vi "Demo_Main-Administrator-an.vi"() -> ()   [LabVIEW 2010]
uses:
  ControlCAN/ControlCAN.llb/DevType.ctl
  ControlCAN/ControlCAN.llb/CAN Channel.ctl
  ControlCAN/ControlCAN.llb/InitFlag.ctl
  ControlCAN/ControlCAN.llb/Mode.ctl
  ControlCAN/ControlCAN.llb/Fliter.ctl
  ControlCAN/ControlCAN.llb/VCI_CAN_OBJ.ctl
  ControlCAN/ControlCAN.llb/VCI_INIT_CONFIG.ctl
  ControlCAN/ControlCAN.llb/Return Val.ctl
  ControlCAN/ControlCAN.lvlib
panel:
  in  "T4":u16
  in  "W4":u16
  in  "W3":u16
  out "W4":u16
  in  "W4_R":bool
  in  "W4_W":bool
  in  "W3_R":bool
  out "W3":u16
  in  "W3_W":bool
  out "W2":u16
  in  "W2_R":bool
  in  "W2_W":bool
  in  "W2":u16
  in  "W1_R":bool
  in  "W1":u16
  out "W1":u16
  in  "W1_W":bool
  in  "电机自动校准":string(combo)="0"
  in  "电机校准_W":bool
  in  "T4_R":bool
  out "T4":u16
  in  "T4_W":bool
  in  "减速度_R":bool
  in  "减速度":dbl format="%#.6f"
  out "减速度_回":dbl format="%#.6f"
  in  "减速度_W":bool
  out "版本号":dbl format="%_3f"
  in  "看门狗周期_R":bool
  in  "看门狗周期":u16
  out "看门狗周期_回":u16
  in  "看门狗周期_W":bool
  in  "看门狗_W":bool
  in  "看门狗":string(combo)="开启"
  in  "监测周期_R":bool
  in  "监测周期":u16
  out "监测周期_回":u16
  in  "监测周期_W":bool
  out "ERRO7":bool
  out "ERRO6":bool
  out "ERRO5":bool
  out "ERRO4":bool
  out "ERRO3":bool
  out "高温":bool
  out "高压":bool
  out "低压":bool
  out "warn7":bool
  out "warn6":bool
  out "warn5":bool
  out "warn4":bool
  out "warn3":bool
  out "高温":bool
  out "warn1":bool
  out "warn0":bool
  out "温度":dbl format="%#.6f"
  out "转速":dbl(graph)
  out "CAN ID":u8 format="%x"
  out "数组":u8[](array[numeric]) format="%x"
  in  "DATA_SAVE_W":bool
  out "T3":u16
  out "T2":u16
  in  "T3_R":bool
  in  "T2_R":bool
  in  "T3_W":bool
  in  "T2_W":bool
  in  "T3":u16
  in  "T2":u16
  in  "T1_R":bool
  in  "T1":u16
  out "T1":u16
  in  "T1_W":bool
  out "Sin":i32
  out "Cosin":i32
  in  "加速度_R":bool
  in  "加速度":dbl format="%#.6f"
  out "加速度_回":dbl format="%#.6f"
  in  "加速度_W":bool
  in  "速度环KI_R":bool
  in  "W_EN_R":bool
  in  "速度环KI":dbl format="%#.6f"
  out "速度环KI_回":dbl format="%#.6f"
  in  "速度环KI_W":bool
  in  "过载诊断使能":i8
  out "功率使能":i8
  in  "W_EN_W":bool
  in  "I_EN_R":bool
  in  "Direction_R":bool
  in  "电流诊断使能":i8
  out "电流使能":i8
  in  "I_EN_W":bool
  in  "方向":u16
  out "方向":i8
  in  "Direction_W":bool
  out "波形图表3":dbl(graph)
  out "波形图表2":dbl(graph)
  out "波形图表1":dbl(graph)
  out "sCnt":u32 caption="处理统计"
  out "模式_回":string(combo)="00"
  in  "模式_R":bool
  in  "设定电流_R":bool
  in  "设定位置_R":bool
  in  "设定速度_R":bool
  in  "存储路径":path
  in  "保存":bool
  out "保存_S":bool
  in  "模式_W":bool
  in  "模式":string(combo)="00"
  in  "设定电流":dbl format="%#.6f"
  out "设定电流_回":dbl format="%#.6f"
  in  "设定电流_W":bool
  in  "设定位置":dbl format="%#.6f"
  out "设定位置_回":dbl format="%#.6f"
  in  "设定位置_W":bool
  in  "设定速度":dbl format="%#.1f"
  out "设定速度_回":dbl format="%#.6f"
  in  "设定速度_W":bool
  in  "监测_W":bool
  in  "监测":string(combo)="30"
  out "电机ID_R":u32
  in  "Clear":bool
  out "Ualfa":dbl format="%#.6f"
  out "Ubate":dbl format="%#.6f"
  out "Uq":dbl format="%#.6f"
  out "Ud":dbl format="%#.6f"
  out "PWM1":u16
  out "PWM2":u16
  out "PWM3":u16
  out "sector":u8
  out "Iqnow":dbl
  out "Idnow":dbl
  out "Ialfa":dbl
  out "Ibeta":dbl
  out "A电流":dbl
  out "C电流":dbl
  out "B电流":dbl
  out "供电电压":dbl
  out "机械角度":dbl format="%.2f"
  out "电气角度":dbl
  out "转速":dbl
  out "CAN STD_ID":u32 format="%x"
  in  "电机ID":string(combo)="00"
  in  "电机ID_W":bool
  out "RecvCnt":u32 caption="接收统计"
  out "SendCnt":u32 caption="发送统计"
  in  "Format":u8(ring) items=["标准帧", "扩展帧"]
  in  "Type":u8(ring) items=["数据帧", "远程帧"]
  in  "Data":string="00 01 02 03 04 05 06 07"
  in  "ID":u32=291 format="0x%x"
  in  "Send":bool
  in  "RcvEnable":bool=TRUE
  out "Open":bool
  in  "Fliter":T1=1 items=["接收所有类型"=1, "只接收标准帧"=2, "只接收扩展帧"=3]
  in  "kBaudRate":u8(ring)=12 caption="波特率" items=["5k bps"=1, "10k bps"=2, "20k bps"=3, "40k bps"=4, "50k bps"=5, "80k bps"=6, "100k bps"=7, "125k bps"=8, "200k bps"=9, "250k bps"=10, "400k bps"=11, "500k bps"=12, "666k bps"=13, "800k bps"=14, "1000k bps"=15, "33.33k bps"=16, "66.66k bps"=17, "83.33k bps"=18]
  in  "Mode":T2 caption="工作模式" items=["正常工作", "仅侦听模式", "自测模式（环回）"]
  in  "InitFlag":T3 caption="初始化参数" items=["使用Flash参数", "使用界面设置参数"]
  in  "AccMask":u32=4294967295 caption="接收屏蔽码" format="%08x"
  in  "AccCode":u32 caption="接收过滤码" format="%08x"
  in  "Close":bool
  in  "Open":bool
  in  "Channel":T4 caption="CAN通道" items=["通道1", "通道2"]
  in  "DevType":T5=3 caption="设备类型" items=["USB-CAN"=2, "USB-CAN2"=3]
  # "发送指令帧包"
  # "CAN\n  ID"
  # "DATA"
  # "DATA"
  # "DATA"
  # "0"
  # "1"
  # "7"
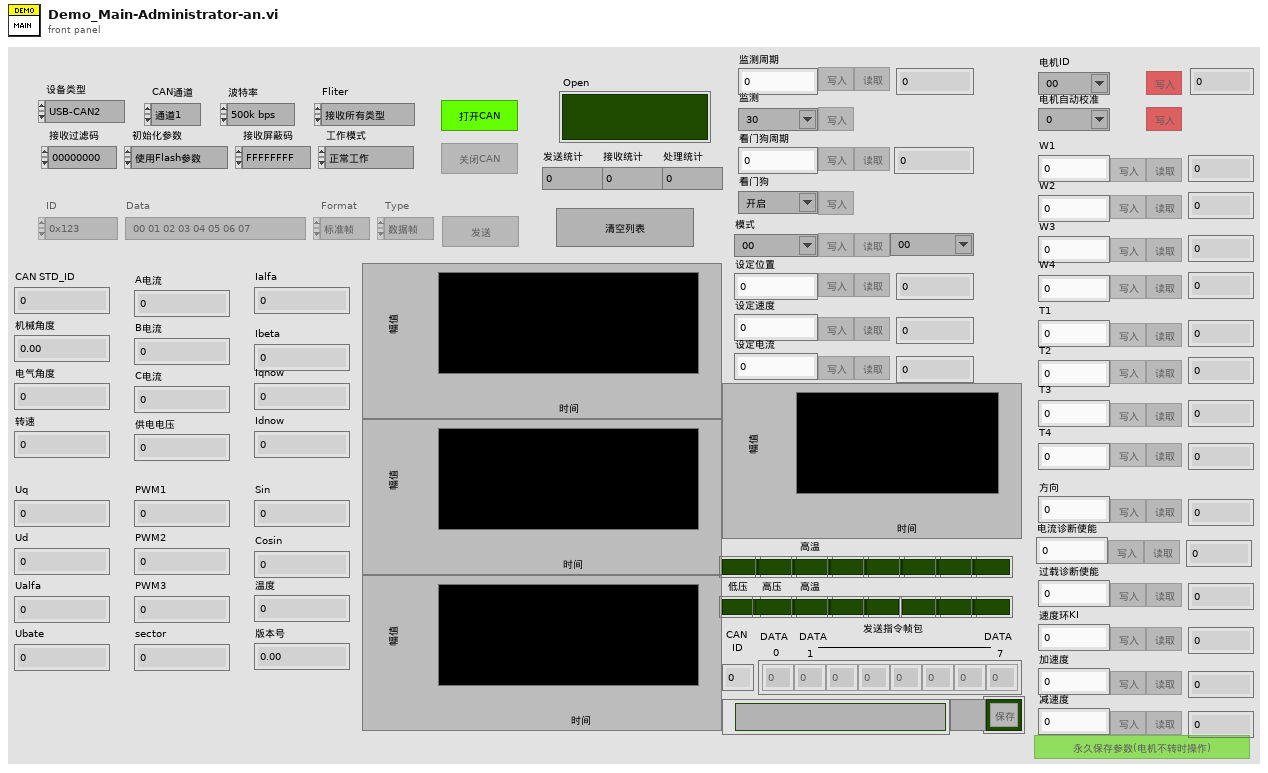
[diagram p1: front panel]
types:
  T1 = typedef "ControlCAN.lvlib/Fliter.ctl" = u8
  T2 = typedef "ControlCAN.lvlib/Mode.ctl" = u8
  T3 = typedef "ControlCAN.lvlib/InitFlag.ctl" = u32
  T4 = typedef "ControlCAN.lvlib/CAN Channel.ctl" = u32
  T5 = typedef "ControlCAN.lvlib/DevType.ctl" = u32
  T6 = typedef "ControlCAN.lvlib/VCI_CAN_OBJ.ctl" = cluster{"ID":u32, "TimeStamp":u32, "TimeFlag":u8, "SendType":u8, "RemoteFlag":u8, "ExternFlag":u8, "DataLen":u8, "Data":u8[], "Reserved":u8[]}
  T7 = cluster{"Type":enum16{"接收", "发送"}, "Channel":T4, "Time":timestamp, "VCI_CAN_OBJ":T6}[]
  T8 = typedef "ControlCAN.lvlib/VCI_INIT_CONFIG.ctl" = cluster{"AccCode":u32, "AccMask":u32, "InitFlag":T3, "Fliter":T1, "Timing0":u8, "Timing1":u8, "Mode":T2}
  T9 = cluster{"DevType":T5, "DevIndex":u32, "CanIndex":T4, "VCI_INIT_CONFIG":T8}
  T10 = typedef "ControlCAN.lvlib/Return Val.ctl" = i32
  T11 = enum16{"open", "replace", "create", "open or create", "replace or create", "replace or create with confirmation"}
  T12 = cluster{"[0]":cluster{"Type":enum16{"接收", "发送"}, "Channel":T4, "Time":timestamp, "VCI_CAN_OBJ":T6}}
  T13 = cluster{"Type":enum16{"接收", "发送"}, "Channel":T4, "Time":timestamp, "VCI_CAN_OBJ":T6}
  T14 = cluster{"Data[0]":u8, "Data[1]":u8, "Data[2]":u8, "Data[3]":u8, "Data[4]":u8, "Data[5]":u8, "Data[6]":u8, "Data[7]":u8}
  T15 = cluster{"Boolean array[0]":bool, "Boolean array[1]":bool, "Boolean array[2]":bool, "Boolean array[3]":bool, "Boolean array[4]":bool, "Boolean array[5]":bool, "Boolean array[6]":bool, "Boolean array[7]":bool}
  T16 = enum32{"invalid app kind", "Development System", "Run Time System", "Student Edition", "Embedded LabVIEW", "Evaluation", "Custom"}
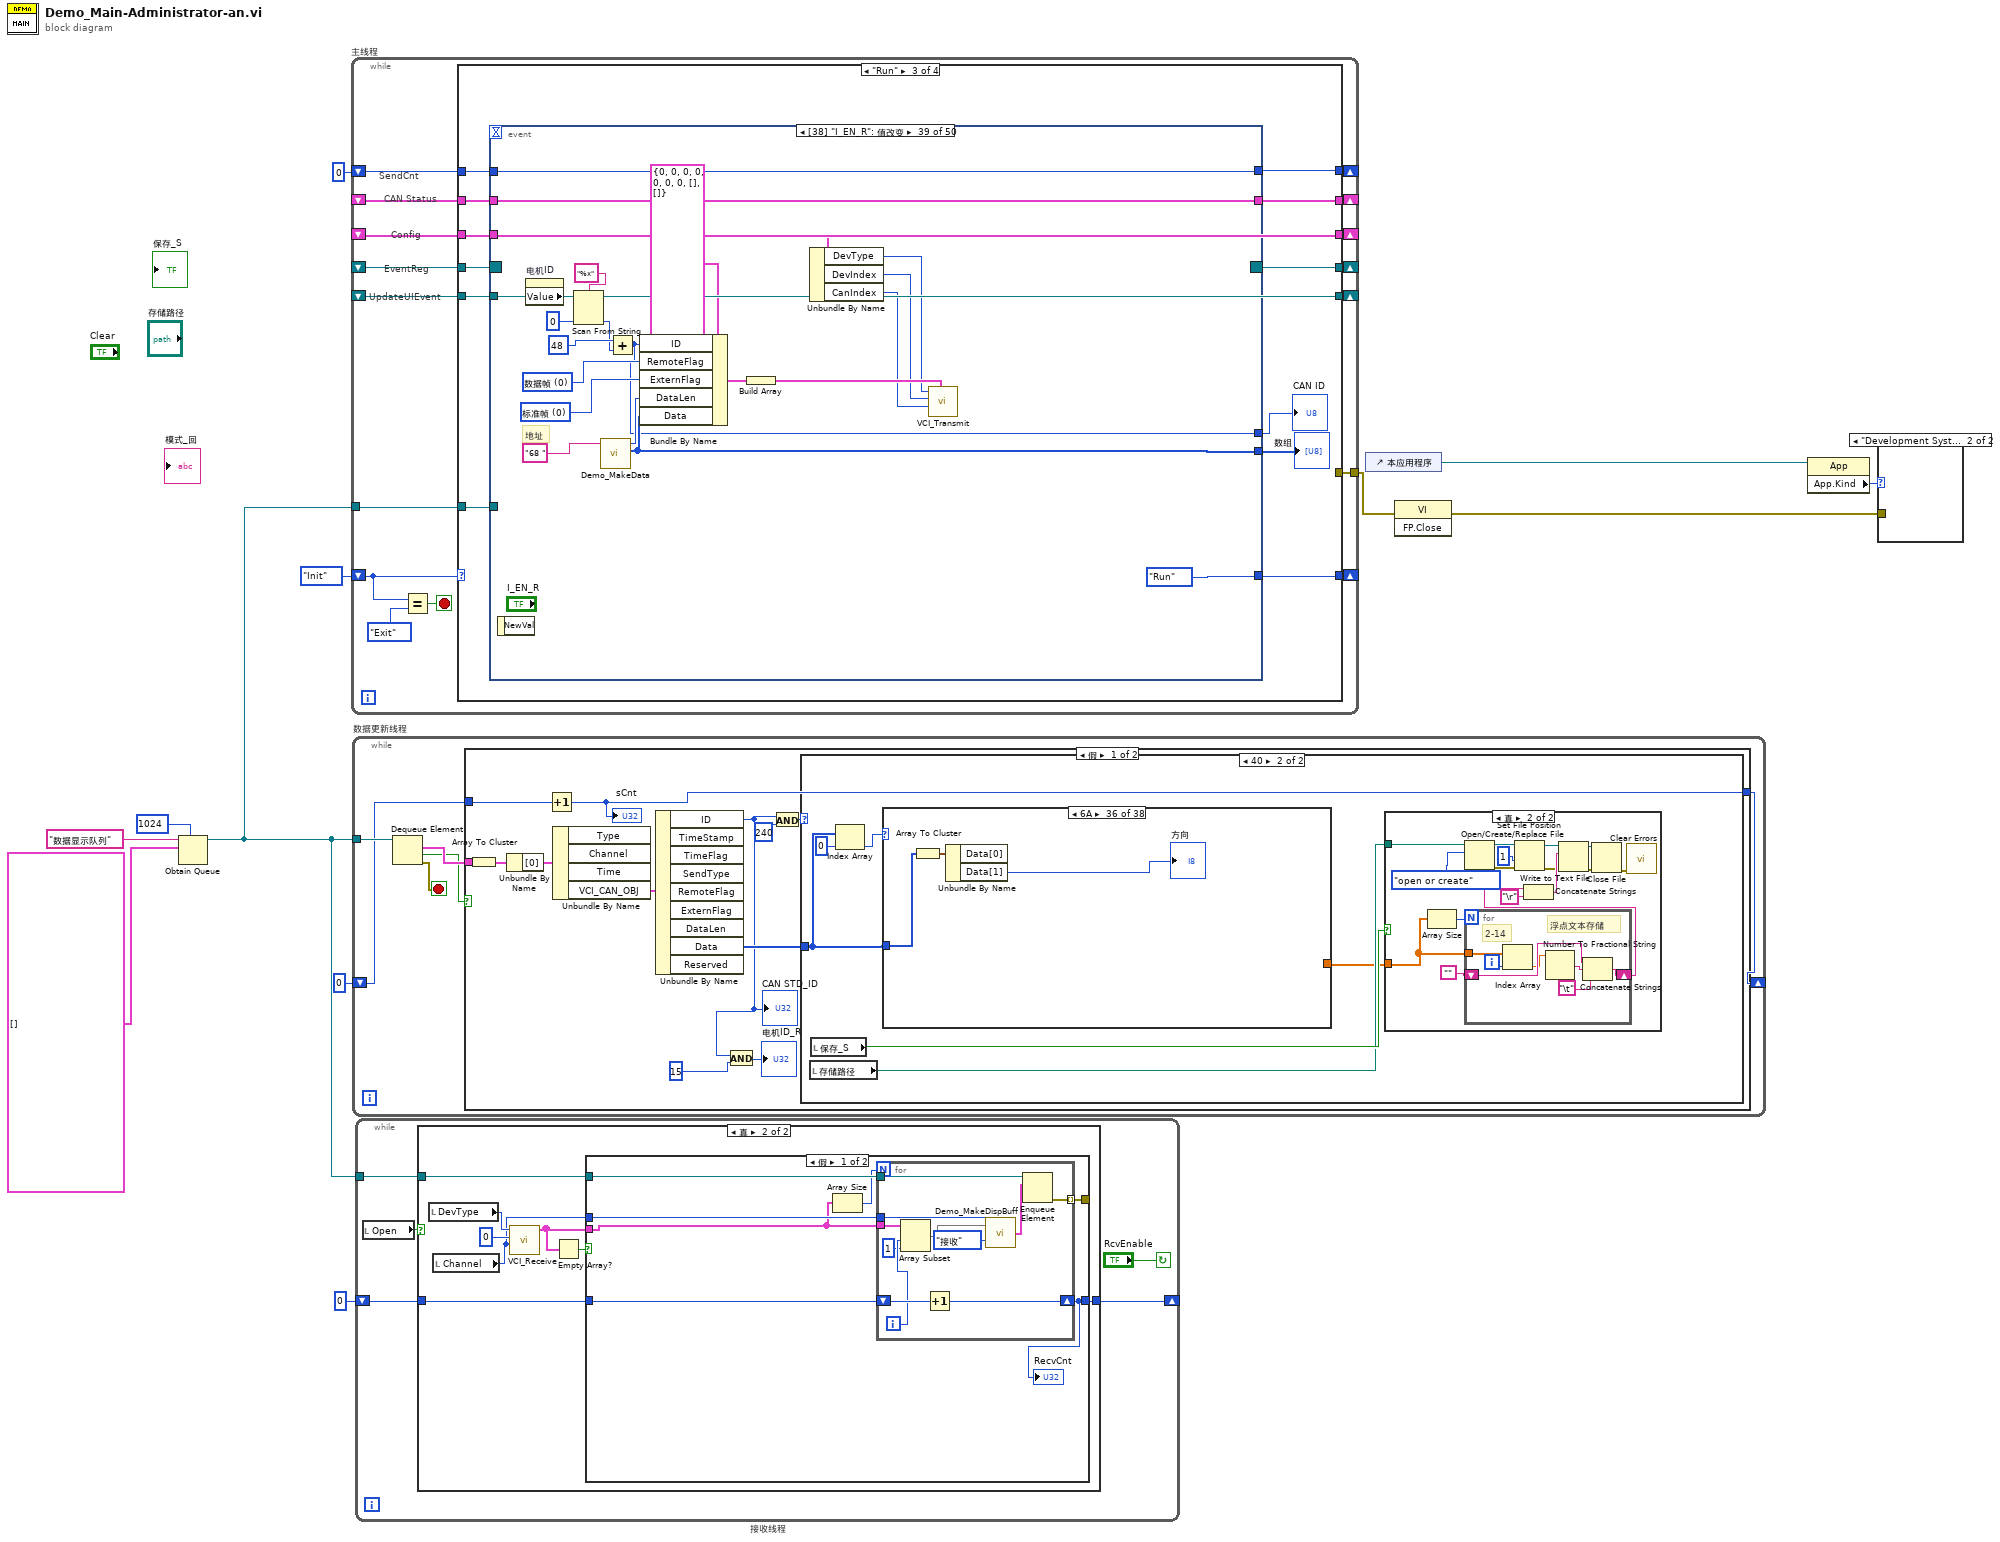
[diagram p0: block diagram]
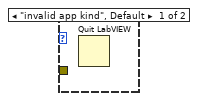
[diagram p2: hidden frame]
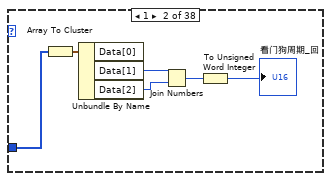
[diagram p6: hidden frame]
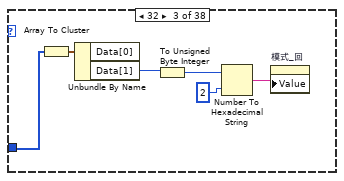
[diagram p7: hidden frame]
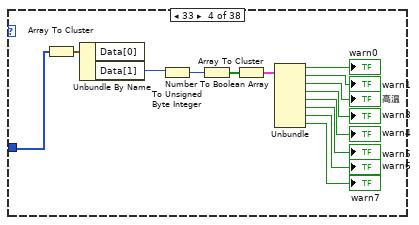
[diagram p8: hidden frame]
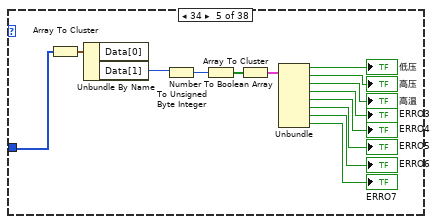
[diagram p9: hidden frame]
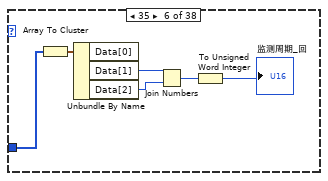
[diagram p10: hidden frame]
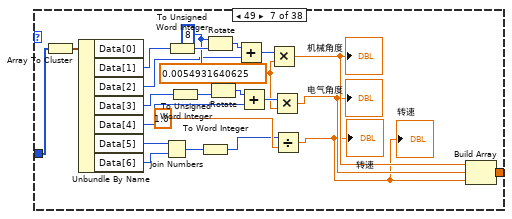
[diagram p11: hidden frame]
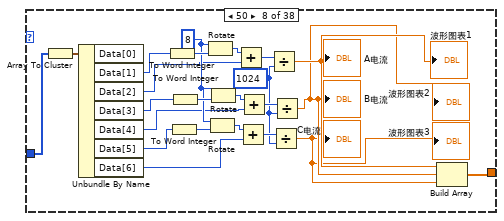
[diagram p12: hidden frame]
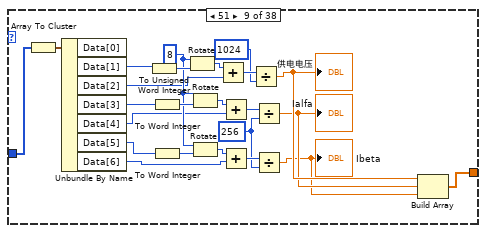
[diagram p13: hidden frame]
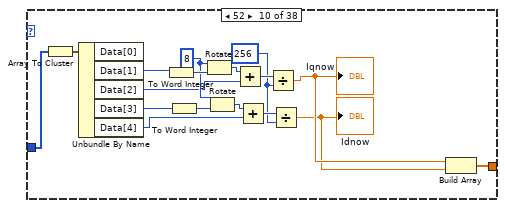
[diagram p14: hidden frame]
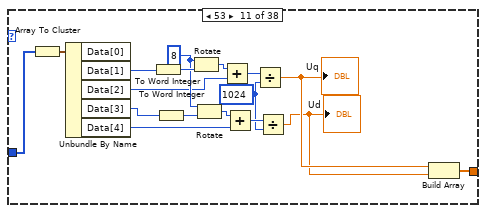
[diagram p15: hidden frame]
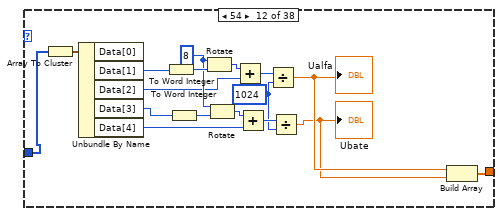
[diagram p16: hidden frame]
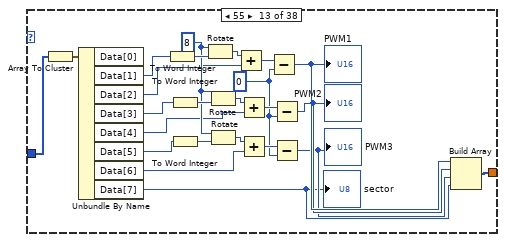
[diagram p17: hidden frame]
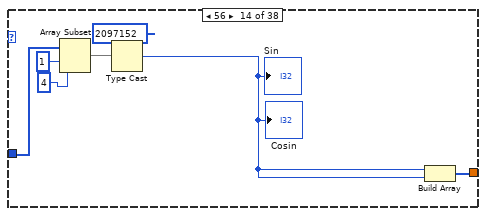
[diagram p18: hidden frame]
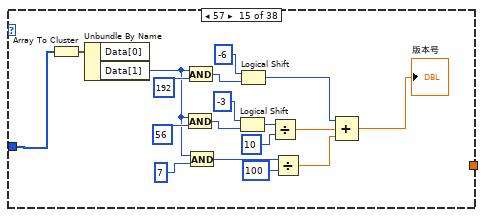
[diagram p19: hidden frame]
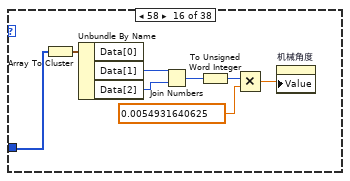
[diagram p20: hidden frame]
diagram:
  n1 = Obtain Queue(max queue size (-1, unlimited)=1024, name (unnamed)="数据显示队列" ("名称（未命名）"), element data type=T7 []) -> (queue out=w9:refnum<queue>)  [unwired: 2 in, 2 out]
  n2 = while "主线程" {
    shift-right: [w24] -> _
    shift-left: enum16{"Init", "Wait", "Run", "Exit"}."Init" -> [w27]
    shift-right: [w25] -> _
    shift-left: _ -> [w26]
    shift-right: [w23] -> _
    shift-left: _ -> [w22]
    tunnel: w9 -> [w21]
    shift-right: [w19] -> _
    shift-left: _ -> [w18]
    shift-right: [w17] -> _
    shift-left: _ -> [w16]
    shift-right: [w14] -> _
    shift-left: u32 0 -> [w15]
    tunnel: [w13] -> w4
    stop <- w28 stop-if-true
    # "CAN Status"
    # "Config"
    # "EventReg"
    # "UpdateUIEvent"
    # "SendCnt"
    n3 = Equal?(x=w27, y=enum16{"Init", "Wait", "Run", "Exit"}."Exit") -> (x = y?=w28:bool)
    n4 = case shown="\"Run\"" w27 {
      tunnel: w26 -> [_ w57 w158 w1251]
      tunnel: [w48 w56 w157 w1251] -> w25
      tunnel: [enum16{"Init", "Wait", "Run", "Exit"}."Wait" w53 w160 enum16{"Init", "Wait", "Run", "Exit"}."Exit"] -> w24
      tunnel: [w44 w54 w156 w1249] -> w23
      tunnel: w22 -> [_ w55 w156 w1249]
      tunnel: w21 -> [_ w52 w159 w1255]
      tunnel: [w36 w51 w154 w1254] -> w19
      tunnel: w18 -> [_ w51 w155 w1254]
      tunnel: [w35 w50 w153 w1252] -> w17
      tunnel: w16 -> [_ w50 w153 w1252]
      tunnel: w15 -> [w33 w49 w152 w1247]
      tunnel: [w33 w49 w151 w1247] -> w14
      tunnel: [_ _ _ errorcluster {"status"=FALSE, "code"=0, "source"=""} ("error constant")] -> w13
      frame "Init", Default {
        w37 = cluster{"CANOpen":bool} {"CANOpen"=FALSE}  # UpdateUI
        w47 = T9 {"DevType"=2, "DevIndex"=0, "CanIndex"=0, "VCI_INIT_CONFIG"={"AccCode"=0, "AccMask"=0, "InitFlag"=0, "Fliter"=0, "Timing0"=0, "Timing1"=0, "Mode"=0}}  # Config
        w48 = cluster{"Open":bool, "SendCnt":u32} {"Open"=FALSE, "SendCnt"=0}  # CAN Status
        n5 = property class="VI"("Front Panel.Closeable"=TRUE ("前面板窗口:可关闭")) -> ()  [unwired: 2 in, 2 out]
        n6 = invoke class="VI" method="Default Vals.Reinit All"() -> ()  [unwired: 3 in, 3 out]
        n7 = call "Demo_GetT0T1.vi"("kBaudRate"="kBaudRate") -> ("Timing0"=w30:u8, "Timing1"=w29:u8)
        n8 = Bundle By Name(cluster=w47, "DevType"="DevType", "CanIndex"="Channel", "VCI_INIT_CONFIG.AccCode"="AccCode", "VCI_INIT_CONFIG.AccMask"="AccMask", "VCI_INIT_CONFIG.InitFlag"="InitFlag", "VCI_INIT_CONFIG.Fliter"="Fliter", "VCI_INIT_CONFIG.Timing0"=w30, "VCI_INIT_CONFIG.Timing1"=w29, "VCI_INIT_CONFIG.Mode"="Mode") -> (w44:T9)
        n9 = local write "RcvEnable"(TRUE ("RcvEnable")) -> ()
        n10 = Create User Event(user event datatype=w37) -> (user event=w35:refnum<user-event>)  [unwired: 1 in, 1 out]
        n11 = register-events(w35) -> (reference out=w36:refnum<event-registration>)  [unwired: 2 in, 1 out]
      }
      frame "Wait" {
        n12 = event shown="[1] 前面板关闭？" {
          selector: _ -> [_ _ _ _ _ _ _ _ _ _]
          dyn-events: _ -> [_ _ _ _ _ _ _ _ _ _]
          timeout: _ -> [_ _ _ _ _ _ _ _ _ _]
          tunnel: w57 -> [w61 w101 w111 w116 w121 w126 w131 w136 w143 w148]
          tunnel: [w60 w101 w111 w116 w121 w126 w131 w136 w143 w148] -> w56
          tunnel: w55 -> [w71 w100 w110 w115 w120 w125 w130 w135 w142 w147]
          tunnel: [w71 w100 w109 w113 w118 w123 w128 w133 w141 w145] -> w54
          tunnel: [w62 enum16{"Init", "Wait", "Run", "Exit"}."Exit" enum16{"Init", "Wait", "Run", "Exit"}."Wait" enum16{"Init", "Wait", "Run", "Exit"}."Wait" enum16{"Init", "Wait", "Run", "Exit"}."Wait" enum16{"Init", "Wait", "Run", "Exit"}."Wait" enum16{"Init", "Wait", "Run", "Exit"}."Wait" enum16{"Init", "Wait", "Run", "Exit"}."Wait" enum16{"Init", "Wait", "Run", "Exit"}."Wait" enum16{"Init", "Wait", "Run", "Exit"}."Wait"] -> w53
          tunnel: w52 -> [_ _ _ _ _ _ _ _ _ _]
          tunnel: w50 -> [w59 _ _ _ _ _ _ _ _ _]
          event "Open": Value Change {
            w65 = T10 1 items=["OK"=1, "ERROR1"=0, "ERROR2"=-1] ("y")
            # "打开CAN的步骤：\n1.Open\n2.Init\n3.Start"
            n13 = event-data() -> ()  [unwired: 2 out]
            n14 = Unbundle By Name(w71) -> ("DevType"=w70:T5, "DevIndex"=w69:u32)
            n15 = call "VCI_OpenDevice.vi"("DevIndex"=w69, "DevType"=w70) -> ("error out"=w66:errorcluster, "Return Val"=w68:T10)  [unwired: 2 in, 6 out]
            n16 = Equal?(x=w68, y=w65) -> (x = y?=w67:bool)
            n17 = case shown="真" w67 {
              tunnel: w66 -> [_ w86]
              tunnel: w71 -> [_ w85]
              tunnel: w65 -> [_ w77]
              tunnel: [_ w76] -> w58
              frame False {
              }
              frame True {
                n18 = Unbundle By Name(w85) -> ("VCI_INIT_CONFIG"=w84:T8, "DevType"=w80:T5, "DevIndex"=w79:u32, "CanIndex"=w78:T4)
                n19 = call "VCI_InitCAN.vi"("VCI_INIT_CONFIG"=w84, "error in (no error)"=w86, "CANIndex"=w78, "DevIndex"=w79, "DevType"=w80) -> ("error out"=w81:errorcluster, "Return Val"=w83:T10)  [unwired: 5 out]
                n20 = Equal?(x=w77, y=w83) -> (x = y?=w82:bool)
                n21 = case shown="真" w82 {
                  tunnel: w81 -> [_ w97]
                  tunnel: w80 -> [_ w96]
                  tunnel: w79 -> [_ w95]
                  tunnel: w78 -> [_ w94]
                  tunnel: w77 -> [_ w92]
                  tunnel: [_ w88] -> w76
                  frame False {
                  }
                  frame True {
                    n22 = call "VCI_StartCAN.vi"("error in (no error)"=w97, "CANIndex"=w94, "DevIndex"=w95, "DevType"=w96) -> ("error out"=w90:errorcluster, "Return Val"=w93:T10)  [unwired: 6 out]
                    n23 = Unbundle By Name(w90) -> ("status"=w87:bool)
                    n24 = Equal?(x=w92, y=w93) -> (x = y?=w91:bool)
                    n25 = Not(x=w87) -> (.not. x?=w89:bool)
                    n26 = And(x=w91, y=w89) -> (x .and. y?=w88:bool)
                  }
                }
              }
            }
            n27 = case shown="真" w58 {
              tunnel: w59 -> [_ w75]
              tunnel: w58 -> [_ w73]
              frame False {
              }
              frame True {
                n28 = Bundle By Name(cluster=cluster{"CANOpen":bool} {"CANOpen"=FALSE} ("事件数据"), "CANOpen"=w73) -> (w72:cluster{"CANOpen":bool})
                n29 = Generate User Event(user event=w75, event data cluster=w72) -> ()  [unwired: 1 in, 2 out]
              }
            }
            n30 = Select(t=enum16{"Init", "Wait", "Run", "Exit"}."Run", s=w58, f=enum16{"Init", "Wait", "Run", "Exit"}."Wait") -> (s? t:f=w62:enum16{"Init", "Wait", "Run", "Exit"})
            n31 = Bundle By Name(cluster=w61, "Open"=w58) -> (w60:cluster{"Open":bool, "SendCnt":u32})
          }
          event Panel Close? {
            n32 = event-data() -> ()  [unwired: 2 out]
            n33 = event-data("Discard?"=TRUE ("放弃？")) -> ()  [unwired: 1 in, 1 out]
          }
          event Value Change {
            w107 = T5 3 items=["USB-CAN"=2, "USB-CAN2"=3] ("y")
            n34 = event-data() -> ("NewVal"=w108:T5)  [unwired: 1 out]
            n35 = Equal?(x=w108, y=w107) -> (x = y?=w106:bool)
            n36 = Bundle By Name(cluster=w110, "DevType"=w108) -> (w109:T9)
            n37 = Select(t=i32[] [] ("禁用项[]"), s=w106, f=i32[] [1] ("禁用项[]")) -> (s? t:f=w105:i32[])
            n38 = property on="Channel" class="Ring (严格)"("Disabled Items []"=w105) -> ()  [unwired: 2 in, 2 out]
          }
          event Value Change {
            n39 = event-data() -> ("NewVal"=w114:T4)  [unwired: 1 out]
            n40 = Bundle By Name(cluster=w115, "CanIndex"=w114) -> (w113:T9)
          }
          event "AccCode": Value Change {
            n41 = event-data() -> ("NewVal"=w119:u32)  [unwired: 1 out]
            n42 = Bundle By Name(cluster=w120, "VCI_INIT_CONFIG.AccCode"=w119) -> (w118:T9)
          }
          event "AccMask": Value Change {
            n43 = event-data() -> ("NewVal"=w124:u32)  [unwired: 1 out]
            n44 = Bundle By Name(cluster=w125, "VCI_INIT_CONFIG.AccMask"=w124) -> (w123:T9)
          }
          event Value Change {
            n45 = event-data() -> ("NewVal"=w129:T3)  [unwired: 1 out]
            n46 = Bundle By Name(cluster=w130, "VCI_INIT_CONFIG.InitFlag"=w129) -> (w128:T9)
          }
          event Value Change {
            n47 = event-data() -> ("NewVal"=w134:T2)  [unwired: 1 out]
            n48 = Bundle By Name(cluster=w135, "VCI_INIT_CONFIG.Mode"=w134) -> (w133:T9)
          }
          event "kBaudRate": Value Change {
            n49 = event-data() -> ("NewVal"=w139:u8)  [unwired: 1 out]
            n50 = call "Demo_GetT0T1.vi"("kBaudRate"=w139) -> ("Timing0"=w138:u8, "Timing1"=w137:u8)
            n51 = Bundle By Name(cluster=w142, "VCI_INIT_CONFIG.Timing0"=w138, "VCI_INIT_CONFIG.Timing1"=w137) -> (w141:T9)
          }
          event Value Change {
            n52 = event-data() -> ("NewVal"=w146:T1)  [unwired: 1 out]
            n53 = Bundle By Name(cluster=w147, "VCI_INIT_CONFIG.Fliter"=w146) -> (w145:T9)
          }
        }
      }
      frame "Run" {
        n54 = event shown="[38] \"I_EN_R\": 值改变" {
          selector: w155 -> [_ _ _ _ _ _ _ _ _ _ _ _ _ _ _ _ _ _ _ _ _ _ _ _ _ _ _ _ _ _ _ _ _ _ _ _ _ _ _ _ _ _ _ _ _ _ _ _ _ _]
          dyn-events: [_ _ _ _ _ _ _ _ _ _ _ _ _ _ _ _ _ _ _ _ _ _ _ _ _ _ _ _ _ _ _ _ _ _ _ _ _ _ _ _ _ _ _ _ _ _ _ _ _ _] -> w154
          timeout: _ -> [_ _ _ _ _ _ _ _ _ _ _ _ _ _ _ _ _ _ _ _ _ _ _ _ _ _ _ _ _ _ _ _ _ _ _ _ _ _ _ _ _ _ _ _ _ _ _ _ _ _]
          tunnel: [enum16{"Init", "Wait", "Run", "Exit"}."Run" enum16{"Init", "Wait", "Run", "Exit"}."Run" enum16{"Init", "Wait", "Run", "Exit"}."Run" enum16{"Init", "Wait", "Run", "Exit"}."Run" enum16{"Init", "Wait", "Run", "Exit"}."Run" enum16{"Init", "Wait", "Run", "Exit"}."Run" enum16{"Init", "Wait", "Run", "Exit"}."Run" enum16{"Init", "Wait", "Run", "Exit"}."Run" enum16{"Init", "Wait", "Run", "Exit"}."Run" enum16{"Init", "Wait", "Run", "Exit"}."Run" enum16{"Init", "Wait", "Run", "Exit"}."Run" enum16{"Init", "Wait", "Run", "Exit"}."Run" enum16{"Init", "Wait", "Run", "Exit"}."Run" enum16{"Init", "Wait", "Run", "Exit"}."Run" enum16{"Init", "Wait", "Run", "Exit"}."Run" enum16{"Init", "Wait", "Run", "Exit"}."Run" enum16{"Init", "Wait", "Run", "Exit"}."Run" enum16{"Init", "Wait", "Run", "Exit"}."Run" enum16{"Init", "Wait", "Run", "Exit"}."Run" enum16{"Init", "Wait", "Run", "Exit"}."Run" enum16{"Init", "Wait", "Run", "Exit"}."Run" enum16{"Init", "Wait", "Run", "Exit"}."Run" enum16{"Init", "Wait", "Run", "Exit"}."Run" enum16{"Init", "Wait", "Run", "Exit"}."Run" enum16{"Init", "Wait", "Run", "Exit"}."Run" enum16{"Init", "Wait", "Run", "Exit"}."Run" enum16{"Init", "Wait", "Run", "Exit"}."Run" enum16{"Init", "Wait", "Run", "Exit"}."Run" enum16{"Init", "Wait", "Run", "Exit"}."Run" enum16{"Init", "Wait", "Run", "Exit"}."Run" enum16{"Init", "Wait", "Run", "Exit"}."Run" enum16{"Init", "Wait", "Run", "Exit"}."Run" enum16{"Init", "Wait", "Run", "Exit"}."Run" enum16{"Init", "Wait", "Run", "Exit"}."Run" enum16{"Init", "Wait", "Run", "Exit"}."Run" enum16{"Init", "Wait", "Run", "Exit"}."Run" enum16{"Init", "Wait", "Run", "Exit"}."Run" enum16{"Init", "Wait", "Run", "Exit"}."Run" enum16{"Init", "Wait", "Run", "Exit"}."Run" enum16{"Init", "Wait", "Run", "Exit"}."Run" enum16{"Init", "Wait", "Run", "Exit"}."Run" enum16{"Init", "Wait", "Run", "Exit"}."Run" enum16{"Init", "Wait", "Run", "Exit"}."Run" enum16{"Init", "Wait", "Run", "Exit"}."Run" enum16{"Init", "Wait", "Run", "Exit"}."Run" enum16{"Init", "Wait", "Run", "Exit"}."Run" enum16{"Init", "Wait", "Run", "Exit"}."Run" enum16{"Init", "Wait", "Run", "Exit"}."Run" enum16{"Init", "Wait", "Run", "Exit"}."Run" w1240] -> w160
          tunnel: w159 -> [_ _ _ _ _ _ _ _ _ _ _ _ _ _ _ _ _ _ _ _ _ _ _ _ _ _ _ _ _ _ _ _ _ _ _ _ _ _ _ _ _ _ _ _ _ _ _ _ _ _]
          tunnel: [w162 w179 w196 w219 w243 w264 w288 w309 w333 w354 w378 w399 w423 w444 w465 w484 w505 w521 w559 w580 w606 w632 w658 w680 w702 w724 w750 w776 w802 w826 w850 w874 w898 w919 w940 w961 w982 w1003 w1024 w1045 w1066 w1087 w1108 w1129 w1150 w1171 w1192 w1220 w1226 w1245] -> w157
          tunnel: w158 -> [w162 w179 w196 w219 w243 w264 w288 w309 w333 w354 w378 w399 w423 w444 w465 w484 w505 w521 w559 w580 w606 w632 w658 w680 w702 w724 w750 w776 w802 w826 w850 w874 w898 w919 w940 w961 w982 w1003 w1024 w1045 w1066 w1087 w1108 w1129 w1150 w1171 w1192 w1220 w1228 w1245]
          tunnel: w156 -> [_ w174 w186 w201 w227 w247 w269 w292 w317 w337 w362 w382 w404 w427 w454 w470 w488 w511 w541 w563 w591 w614 w640 w664 w685 w707 w729 w755 w781 w807 w831 w855 w879 w902 w923 w944 w965 w986 w1007 w1029 w1049 w1070 w1091 w1112 w1133 w1154 w1175 _ w1233 _]
          tunnel: w153 -> [_ _ _ _ _ _ _ _ _ _ _ _ _ _ _ _ _ _ _ _ _ _ _ _ _ _ _ _ _ _ _ _ _ _ _ _ _ _ _ _ _ _ _ _ _ _ _ _ w1225 _]
          tunnel: w152 -> [w161 w167 w195 w218 w242 w263 w287 w308 w332 w353 w377 w398 w422 w443 w464 w483 w504 w520 w558 w579 w605 w631 w657 w679 w701 w723 w749 w775 w801 w825 w849 w873 w897 w918 w939 w960 w981 w1002 w1023 w1044 w1065 w1086 w1107 w1128 w1149 w1170 w1191 w1219 w1221 w1239]
          tunnel: [w161 w166 w195 w218 w242 w263 w287 w308 w332 w353 w377 w398 w422 w443 w464 w483 w504 w520 w558 w579 w605 w631 w657 w679 w701 w723 w749 w775 w801 w825 w849 w873 w897 w918 w939 w960 w981 w1002 w1023 w1044 w1065 w1086 w1107 w1128 w1149 w1170 w1191 w1219 w1221 w1239] -> w151
          tunnel: [_ _ w182 w199 w224 w245 w266 w290 w311 w335 w355 w380 w402 w425 w446 w468 w486 w507 w539 w561 w582 w608 w634 w662 w683 w705 w726 w752 w779 w804 w828 w852 w877 w900 w921 w942 w963 w984 w1005 w1027 w1047 w1068 w1089 w1110 w1131 w1152 w1173 _ _ _] -> w150
          tunnel: [_ _ w181 w200 w226 w246 w267 w291 w316 w336 w361 w381 w403 w426 w445 w469 w487 w510 w538 w560 w581 w607 w633 w661 w682 w704 w725 w751 w778 w803 w827 w851 w878 w899 w920 w941 w962 w983 w1004 w1026 w1046 w1067 w1090 w1109 w1130 w1151 w1174 _ _ _] -> w149
          event Timeout {
            n55 = event-data() -> ()  [unwired: 3 out]
          }
          event "Send": Value Change {
            n56 = event-data() -> ()  [unwired: 2 out]
            n57 = Increment(x=w167) -> (x+1=w166:u32)
            "SendCnt" <- w166
            n58 = call "Demo_MakeData.vi"("DataString"="Data") -> ("Data"=w169:u8[], "DataLen"=w170:u8)  [unwired: 9 out]
            n59 = Bundle By Name(cluster=T6 {"ID"=0, "TimeStamp"=0, "TimeFlag"=0, "SendType"=0, "RemoteFlag"=0, "ExternFlag"=0, "DataLen"=0, "Data"=[], "Reserved"=[]} ("Send"), "ID"="ID", "RemoteFlag"="Type", "ExternFlag"="Format", "DataLen"=w170, "Data"=w169) -> (w164:T6)
            n60 = Build Array(w164) -> (w165:T6[])
            n61 = Unbundle By Name(w174) -> ("DevType"=w173:T5, "DevIndex"=w172:u32, "CanIndex"=w168:T4)
            n62 = call "VCI_Transmit.vi"("Buffer"=w165, "CANIndex"=w168, "DevIndex"=w172, "DevType"=w173) -> ()  [unwired: 1 in, 7 out]
          }
          event "电机ID_W": Value Change {
            w185 = u8 0 items=["数据帧", "遥控帧"]
            w181 = u32 138
            w184 = u8 0 items=["标准帧", "扩展帧"]
            n63 = event-data() -> ()  [unwired: 2 out]
            n64 = call "Demo_MakeData.vi"("DataString"="电机ID") -> ("Data"=w182:u8[], "DataLen"=w190:u8)  [unwired: 9 out]
            n65 = Bundle By Name(cluster=T6 {"ID"=0, "TimeStamp"=0, "TimeFlag"=0, "SendType"=0, "RemoteFlag"=0, "ExternFlag"=0, "DataLen"=0, "Data"=[], "Reserved"=[]} ("Send"), "ID"=w181, "RemoteFlag"=w185, "ExternFlag"=w184, "DataLen"=w190, "Data"=w182) -> (w187:T6)
            n66 = Build Array(w187) -> (w188:T6[])
            n67 = Unbundle By Name(w186) -> ("DevType"=w192:T5, "DevIndex"=w191:u32, "CanIndex"=w189:T4)
            n68 = call "VCI_Transmit.vi"("Buffer"=w188, "CANIndex"=w189, "DevIndex"=w191, "DevType"=w192) -> ()  [unwired: 1 in, 7 out]
          }
          event "电机校准_W": Value Change {
            w216 = u8 0 items=["数据帧", "遥控帧"]
            w217 = u8 0 items=["标准帧", "扩展帧"]
            # "地址"
            n69 = event-data() -> ()  [unwired: 2 out]
            n70 = property on="电机ID" class="CmbBox"() -> ("Value"=w207:string)  [unwired: 2 in, 2 out]
            n71 = Concatenate Strings("20 ", "AA 01 02 03 04 05 55") -> (w203:string)
            n72 = Scan From String(format string="%x" ("格式字符串"), input string=w207, default 1=u8 0) -> (output 1=w204:u8)  [unwired: 2 in, 3 out]
            n73 = call "Demo_MakeData.vi"("DataString"=w203) -> ("Data"=w199:u8[], "DataLen"=w212:u8)  [unwired: 9 out]
            n74 = Add(x=u32 16, y=w204) -> (x+y=w200:u32)
            n75 = Bundle By Name(cluster=T6 {"ID"=0, "TimeStamp"=0, "TimeFlag"=0, "SendType"=0, "RemoteFlag"=0, "ExternFlag"=0, "DataLen"=0, "Data"=[], "Reserved"=[]} ("Send"), "ID"=w200, "RemoteFlag"=w216, "ExternFlag"=w217, "DataLen"=w212, "Data"=w199) -> (w215:T6)
            n76 = Build Array(w215) -> (w214:T6[])
            n77 = Unbundle By Name(w201) -> ("DevType"=w210:T5, "DevIndex"=w211:u32, "CanIndex"=w213:T4)
            n78 = call "VCI_Transmit.vi"("Buffer"=w214, "CANIndex"=w213, "DevIndex"=w211, "DevType"=w210) -> ()  [unwired: 1 in, 7 out]
          }
          event "W1_W": Value Change {
            w239 = u8 0 items=["数据帧", "遥控帧"]
            w240 = u8 0 items=["标准帧", "扩展帧"]
            # "索引地址"
            n79 = event-data() -> ()  [unwired: 2 out]
            n80 = property on="电机ID" class="CmbBox"() -> ("Value"=w231:string)  [unwired: 2 in, 2 out]
            n81 = Scan From String(format string="%x" ("格式字符串"), input string=w231, default 1=u8 0) -> (output 1=w228:u8)  [unwired: 2 in, 3 out]
            n82 = Add(x=u32 16, y=w228) -> (x+y=w226:u32)
            n83 = Split Number(x="W1") -> (hi(x)=w222:u8, lo(x)=w221:u8)
            n84 = Build Array(u8 96, w222, w221) -> (w224:u8[])
            n85 = Bundle By Name(cluster=T6 {"ID"=0, "TimeStamp"=0, "TimeFlag"=0, "SendType"=0, "RemoteFlag"=0, "ExternFlag"=0, "DataLen"=0, "Data"=[], "Reserved"=[]} ("Send"), "ID"=w226, "RemoteFlag"=w239, "ExternFlag"=w240, "DataLen"=u8 3, "Data"=w224) -> (w238:T6)
            n86 = Build Array(w238) -> (w237:T6[])
            n87 = Unbundle By Name(w227) -> ("DevType"=w234:T5, "DevIndex"=w235:u32, "CanIndex"=w236:T4)
            n88 = call "VCI_Transmit.vi"("Buffer"=w237, "CANIndex"=w236, "DevIndex"=w235, "DevType"=w234) -> ()  [unwired: 1 in, 7 out]
          }
          event "W1_R": Value Change {
            w250 = u8 0 items=["数据帧", "遥控帧"]
            w249 = u8 0 items=["标准帧", "扩展帧"]
            # "地址"
            n89 = event-data() -> ()  [unwired: 2 out]
            n90 = property on="电机ID" class="CmbBox"() -> ("Value"=w259:string)  [unwired: 2 in, 2 out]
            n91 = Scan From String(format string="%x" ("格式字符串"), input string=w259, default 1=u8 0) -> (output 1=w262:u8)  [unwired: 2 in, 3 out]
            n92 = call "Demo_MakeData.vi"("DataString"="60") -> ("Data"=w245:u8[], "DataLen"=w254:u8)  [unwired: 9 out]
            n93 = Add(x=u32 48, y=w262) -> (x+y=w246:u32)
            n94 = Bundle By Name(cluster=T6 {"ID"=0, "TimeStamp"=0, "TimeFlag"=0, "SendType"=0, "RemoteFlag"=0, "ExternFlag"=0, "DataLen"=0, "Data"=[], "Reserved"=[]} ("Send"), "ID"=w246, "RemoteFlag"=w250, "ExternFlag"=w249, "DataLen"=w254, "Data"=w245) -> (w251:T6)
            n95 = Build Array(w251) -> (w252:T6[])
            n96 = Unbundle By Name(w247) -> ("DevType"=w256:T5, "DevIndex"=w255:u32, "CanIndex"=w253:T4)
            n97 = call "VCI_Transmit.vi"("Buffer"=w252, "CANIndex"=w253, "DevIndex"=w255, "DevType"=w256) -> ()  [unwired: 1 in, 7 out]
          }
          event "W2_W": Value Change {
            w281 = u8 0 items=["数据帧", "遥控帧"]
            w282 = u8 0 items=["标准帧", "扩展帧"]
            # "索引地址"
            n98 = event-data() -> ()  [unwired: 2 out]
            n99 = property on="电机ID" class="CmbBox"() -> ("Value"=w273:string)  [unwired: 2 in, 2 out]
            n100 = Scan From String(format string="%x" ("格式字符串"), input string=w273, default 1=u8 0) -> (output 1=w270:u8)  [unwired: 2 in, 3 out]
            n101 = Split Number(x="W2") -> (hi(x)=w285:u8, lo(x)=w286:u8)
            n102 = Add(x=u32 16, y=w270) -> (x+y=w267:u32)
            n103 = Build Array(u8 97, w285, w286) -> (w266:u8[])
            n104 = Bundle By Name(cluster=T6 {"ID"=0, "TimeStamp"=0, "TimeFlag"=0, "SendType"=0, "RemoteFlag"=0, "ExternFlag"=0, "DataLen"=0, "Data"=[], "Reserved"=[]} ("Send"), "ID"=w267, "RemoteFlag"=w281, "ExternFlag"=w282, "DataLen"=u8 3, "Data"=w266) -> (w280:T6)
            n105 = Build Array(w280) -> (w279:T6[])
            n106 = Unbundle By Name(w269) -> ("DevType"=w276:T5, "DevIndex"=w277:u32, "CanIndex"=w278:T4)
            n107 = call "VCI_Transmit.vi"("Buffer"=w279, "CANIndex"=w278, "DevIndex"=w277, "DevType"=w276) -> ()  [unwired: 1 in, 7 out]
          }
          event "W2_R": Value Change {
            w295 = u8 0 items=["数据帧", "遥控帧"]
            w294 = u8 0 items=["标准帧", "扩展帧"]
            # "地址"
            n108 = event-data() -> ()  [unwired: 2 out]
            n109 = property on="电机ID" class="CmbBox"() -> ("Value"=w304:string)  [unwired: 2 in, 2 out]
            n110 = Scan From String(format string="%x" ("格式字符串"), input string=w304, default 1=u8 0) -> (output 1=w307:u8)  [unwired: 2 in, 3 out]
            n111 = call "Demo_MakeData.vi"("DataString"="61 ") -> ("Data"=w290:u8[], "DataLen"=w299:u8)  [unwired: 9 out]
            n112 = Add(x=u32 48, y=w307) -> (x+y=w291:u32)
            n113 = Bundle By Name(cluster=T6 {"ID"=0, "TimeStamp"=0, "TimeFlag"=0, "SendType"=0, "RemoteFlag"=0, "ExternFlag"=0, "DataLen"=0, "Data"=[], "Reserved"=[]} ("Send"), "ID"=w291, "RemoteFlag"=w295, "ExternFlag"=w294, "DataLen"=w299, "Data"=w290) -> (w296:T6)
            n114 = Build Array(w296) -> (w297:T6[])
            n115 = Unbundle By Name(w292) -> ("DevType"=w301:T5, "DevIndex"=w300:u32, "CanIndex"=w298:T4)
            n116 = call "VCI_Transmit.vi"("Buffer"=w297, "CANIndex"=w298, "DevIndex"=w300, "DevType"=w301) -> ()  [unwired: 1 in, 7 out]
          }
          event "W3_W": Value Change {
            w320 = u8 0 items=["数据帧", "遥控帧"]
            w319 = u8 0 items=["标准帧", "扩展帧"]
            # "索引地址"
            n117 = event-data() -> ()  [unwired: 2 out]
            n118 = property on="电机ID" class="CmbBox"() -> ("Value"=w328:string)  [unwired: 2 in, 2 out]
            n119 = Scan From String(format string="%x" ("格式字符串"), input string=w328, default 1=u8 0) -> (output 1=w331:u8)  [unwired: 2 in, 3 out]
            n120 = Split Number(x="W3") -> (hi(x)=w313:u8, lo(x)=w314:u8)
            n121 = Add(x=u32 16, y=w331) -> (x+y=w316:u32)
            n122 = Build Array(u8 98, w313, w314) -> (w311:u8[])
            n123 = Bundle By Name(cluster=T6 {"ID"=0, "TimeStamp"=0, "TimeFlag"=0, "SendType"=0, "RemoteFlag"=0, "ExternFlag"=0, "DataLen"=0, "Data"=[], "Reserved"=[]} ("Send"), "ID"=w316, "RemoteFlag"=w320, "ExternFlag"=w319, "DataLen"=u8 3, "Data"=w311) -> (w321:T6)
            n124 = Build Array(w321) -> (w322:T6[])
            n125 = Unbundle By Name(w317) -> ("DevType"=w325:T5, "DevIndex"=w324:u32, "CanIndex"=w323:T4)
            n126 = call "VCI_Transmit.vi"("Buffer"=w322, "CANIndex"=w323, "DevIndex"=w324, "DevType"=w325) -> ()  [unwired: 1 in, 7 out]
          }
          event "W3_R": Value Change {
            w340 = u8 0 items=["数据帧", "遥控帧"]
            w339 = u8 0 items=["标准帧", "扩展帧"]
            # "地址"
            n127 = event-data() -> ()  [unwired: 2 out]
            n128 = property on="电机ID" class="CmbBox"() -> ("Value"=w349:string)  [unwired: 2 in, 2 out]
            n129 = Scan From String(format string="%x" ("格式字符串"), input string=w349, default 1=u8 0) -> (output 1=w352:u8)  [unwired: 2 in, 3 out]
            n130 = call "Demo_MakeData.vi"("DataString"="62") -> ("Data"=w335:u8[], "DataLen"=w344:u8)  [unwired: 9 out]
            n131 = Add(x=u32 48, y=w352) -> (x+y=w336:u32)
            n132 = Bundle By Name(cluster=T6 {"ID"=0, "TimeStamp"=0, "TimeFlag"=0, "SendType"=0, "RemoteFlag"=0, "ExternFlag"=0, "DataLen"=0, "Data"=[], "Reserved"=[]} ("Send"), "ID"=w336, "RemoteFlag"=w340, "ExternFlag"=w339, "DataLen"=w344, "Data"=w335) -> (w341:T6)
            n133 = Build Array(w341) -> (w342:T6[])
            n134 = Unbundle By Name(w337) -> ("DevType"=w346:T5, "DevIndex"=w345:u32, "CanIndex"=w343:T4)
            n135 = call "VCI_Transmit.vi"("Buffer"=w342, "CANIndex"=w343, "DevIndex"=w345, "DevType"=w346) -> ()  [unwired: 1 in, 7 out]
          }
          event "W4_W": Value Change {
            w374 = u8 0 items=["数据帧", "遥控帧"]
            w375 = u8 0 items=["标准帧", "扩展帧"]
            # "索引地址"
            n136 = event-data() -> ()  [unwired: 2 out]
            n137 = property on="电机ID" class="CmbBox"() -> ("Value"=w366:string)  [unwired: 2 in, 2 out]
            n138 = Scan From String(format string="%x" ("格式字符串"), input string=w366, default 1=u8 0) -> (output 1=w363:u8)  [unwired: 2 in, 3 out]
            n139 = Split Number(x="W4") -> (hi(x)=w358:u8, lo(x)=w359:u8)
            n140 = Add(x=u32 16, y=w363) -> (x+y=w361:u32)
            n141 = Build Array(u8 99, w358, w359) -> (w355:u8[])
            n142 = Bundle By Name(cluster=T6 {"ID"=0, "TimeStamp"=0, "TimeFlag"=0, "SendType"=0, "RemoteFlag"=0, "ExternFlag"=0, "DataLen"=0, "Data"=[], "Reserved"=[]} ("Send"), "ID"=w361, "RemoteFlag"=w374, "ExternFlag"=w375, "DataLen"=u8 3, "Data"=w355) -> (w373:T6)
            n143 = Build Array(w373) -> (w372:T6[])
            n144 = Unbundle By Name(w362) -> ("DevType"=w369:T5, "DevIndex"=w370:u32, "CanIndex"=w371:T4)
            n145 = call "VCI_Transmit.vi"("Buffer"=w372, "CANIndex"=w371, "DevIndex"=w370, "DevType"=w369) -> ()  [unwired: 1 in, 7 out]
          }
          event "W4_R": Value Change {
            w385 = u8 0 items=["数据帧", "遥控帧"]
            w384 = u8 0 items=["标准帧", "扩展帧"]
            # "地址"
            n146 = event-data() -> ()  [unwired: 2 out]
            n147 = property on="电机ID" class="CmbBox"() -> ("Value"=w394:string)  [unwired: 2 in, 2 out]
            n148 = Scan From String(format string="%x" ("格式字符串"), input string=w394, default 1=u8 0) -> (output 1=w397:u8)  [unwired: 2 in, 3 out]
            n149 = call "Demo_MakeData.vi"("DataString"="63 ") -> ("Data"=w380:u8[], "DataLen"=w389:u8)  [unwired: 9 out]
            n150 = Add(x=u32 48, y=w397) -> (x+y=w381:u32)
            n151 = Bundle By Name(cluster=T6 {"ID"=0, "TimeStamp"=0, "TimeFlag"=0, "SendType"=0, "RemoteFlag"=0, "ExternFlag"=0, "DataLen"=0, "Data"=[], "Reserved"=[]} ("Send"), "ID"=w381, "RemoteFlag"=w385, "ExternFlag"=w384, "DataLen"=w389, "Data"=w380) -> (w386:T6)
            n152 = Build Array(w386) -> (w387:T6[])
            n153 = Unbundle By Name(w382) -> ("DevType"=w391:T5, "DevIndex"=w390:u32, "CanIndex"=w388:T4)
            n154 = call "VCI_Transmit.vi"("Buffer"=w387, "CANIndex"=w388, "DevIndex"=w390, "DevType"=w391) -> ()  [unwired: 1 in, 7 out]
          }
          event "监测周期_W": Value Change {
            w416 = u8 0 items=["数据帧", "遥控帧"]
            w417 = u8 0 items=["标准帧", "扩展帧"]
            # "索引地址"
            n155 = event-data() -> ()  [unwired: 2 out]
            n156 = property on="电机ID" class="CmbBox"() -> ("Value"=w408:string)  [unwired: 2 in, 2 out]
            n157 = Scan From String(format string="%x" ("格式字符串"), input string=w408, default 1=u8 0) -> (output 1=w405:u8)  [unwired: 2 in, 3 out]
            n158 = Split Number(x="监测周期") -> (hi(x)=w420:u8, lo(x)=w421:u8)
            n159 = Add(x=u32 16, y=w405) -> (x+y=w403:u32)
            n160 = Build Array(u8 35, w420, w421) -> (w402:u8[])
            n161 = Bundle By Name(cluster=T6 {"ID"=0, "TimeStamp"=0, "TimeFlag"=0, "SendType"=0, "RemoteFlag"=0, "ExternFlag"=0, "DataLen"=0, "Data"=[], "Reserved"=[]} ("Send"), "ID"=w403, "RemoteFlag"=w416, "ExternFlag"=w417, "DataLen"=u8 3, "Data"=w402) -> (w415:T6)
            n162 = Build Array(w415) -> (w414:T6[])
            n163 = Unbundle By Name(w404) -> ("DevType"=w411:T5, "DevIndex"=w412:u32, "CanIndex"=w413:T4)
            n164 = call "VCI_Transmit.vi"("Buffer"=w414, "CANIndex"=w413, "DevIndex"=w412, "DevType"=w411) -> ()  [unwired: 1 in, 7 out]
          }
          event "监测周期_R": Value Change {
            w440 = u8 0 items=["数据帧", "遥控帧"]
            w441 = u8 0 items=["标准帧", "扩展帧"]
            # "地址"
            n165 = event-data() -> ()  [unwired: 2 out]
            n166 = property on="电机ID" class="CmbBox"() -> ("Value"=w431:string)  [unwired: 2 in, 2 out]
            n167 = Scan From String(format string="%x" ("格式字符串"), input string=w431, default 1=u8 0) -> (output 1=w428:u8)  [unwired: 2 in, 3 out]
            n168 = call "Demo_MakeData.vi"("DataString"="23 ") -> ("Data"=w425:u8[], "DataLen"=w436:u8)  [unwired: 9 out]
            n169 = Add(x=u32 48, y=w428) -> (x+y=w426:u32)
            n170 = Bundle By Name(cluster=T6 {"ID"=0, "TimeStamp"=0, "TimeFlag"=0, "SendType"=0, "RemoteFlag"=0, "ExternFlag"=0, "DataLen"=0, "Data"=[], "Reserved"=[]} ("Send"), "ID"=w426, "RemoteFlag"=w440, "ExternFlag"=w441, "DataLen"=w436, "Data"=w425) -> (w439:T6)
            n171 = Build Array(w439) -> (w438:T6[])
            n172 = Unbundle By Name(w427) -> ("DevType"=w434:T5, "DevIndex"=w435:u32, "CanIndex"=w437:T4)
            n173 = call "VCI_Transmit.vi"("Buffer"=w438, "CANIndex"=w437, "DevIndex"=w435, "DevType"=w434) -> ()  [unwired: 1 in, 7 out]
          }
          event "监测_W": Value Change {
            w462 = u8 0 items=["数据帧", "遥控帧"]
            w463 = u8 0 items=["标准帧", "扩展帧"]
            # "地址"
            n174 = event-data() -> ()  [unwired: 2 out]
            n175 = property on="电机ID" class="CmbBox"() -> ("Value"=w451:string)  [unwired: 2 in, 2 out]
            n176 = Scan From String(format string="%x" ("格式字符串"), input string=w451, default 1=u8 0) -> (output 1=w448:u8)  [unwired: 2 in, 3 out]
            n177 = call "Demo_MakeData.vi"("DataString"="监测") -> ("Data"=w446:u8[], "DataLen"=w458:u8)  [unwired: 9 out]
            n178 = Add(x=u32 48, y=w448) -> (x+y=w445:u32)
            n179 = Bundle By Name(cluster=T6 {"ID"=0, "TimeStamp"=0, "TimeFlag"=0, "SendType"=0, "RemoteFlag"=0, "ExternFlag"=0, "DataLen"=0, "Data"=[], "Reserved"=[]} ("Send"), "ID"=w445, "RemoteFlag"=w462, "ExternFlag"=w463, "DataLen"=w458, "Data"=w446) -> (w461:T6)
            n180 = Build Array(w461) -> (w460:T6[])
            n181 = Unbundle By Name(w454) -> ("DevType"=w456:T5, "DevIndex"=w457:u32, "CanIndex"=w459:T4)
            n182 = call "VCI_Transmit.vi"("Buffer"=w460, "CANIndex"=w459, "DevIndex"=w457, "DevType"=w456) -> ()  [unwired: 1 in, 7 out]
          }
          event "看门狗周期_W": Value Change {
            w476 = u8 0 items=["数据帧", "遥控帧"]
            w475 = u8 0 items=["标准帧", "扩展帧"]
            w469 = u32 138
            # "索引地址"
            n183 = event-data() -> ()  [unwired: 2 out]
            n184 = Split Number(x="看门狗周期") -> (hi(x)=w472:u8, lo(x)=w471:u8)
            n185 = Build Array(u8 1, w472, w471) -> (w468:u8[])
            n186 = Bundle By Name(cluster=T6 {"ID"=0, "TimeStamp"=0, "TimeFlag"=0, "SendType"=0, "RemoteFlag"=0, "ExternFlag"=0, "DataLen"=0, "Data"=[], "Reserved"=[]} ("Send"), "ID"=w469, "RemoteFlag"=w476, "ExternFlag"=w475, "DataLen"=u8 3, "Data"=w468) -> (w477:T6)
            n187 = Build Array(w477) -> (w478:T6[])
            n188 = Unbundle By Name(w470) -> ("DevType"=w481:T5, "DevIndex"=w480:u32, "CanIndex"=w479:T4)
            n189 = call "VCI_Transmit.vi"("Buffer"=w478, "CANIndex"=w479, "DevIndex"=w480, "DevType"=w481) -> ()  [unwired: 1 in, 7 out]
          }
          event "看门狗周期_R": Value Change {
            w491 = u8 0 items=["数据帧", "遥控帧"]
            w490 = u8 0 items=["标准帧", "扩展帧"]
            # "地址"
            n190 = event-data() -> ()  [unwired: 2 out]
            n191 = property on="电机ID" class="CmbBox"() -> ("Value"=w500:string)  [unwired: 2 in, 2 out]
            n192 = Scan From String(format string="%x" ("格式字符串"), input string=w500, default 1=u8 0) -> (output 1=w503:u8)  [unwired: 2 in, 3 out]
            n193 = call "Demo_MakeData.vi"("DataString"="01") -> ("Data"=w486:u8[], "DataLen"=w495:u8)  [unwired: 9 out]
            n194 = Add(x=u32 48, y=w503) -> (x+y=w487:u32)
            n195 = Bundle By Name(cluster=T6 {"ID"=0, "TimeStamp"=0, "TimeFlag"=0, "SendType"=0, "RemoteFlag"=0, "ExternFlag"=0, "DataLen"=0, "Data"=[], "Reserved"=[]} ("Send"), "ID"=w487, "RemoteFlag"=w491, "ExternFlag"=w490, "DataLen"=w495, "Data"=w486) -> (w492:T6)
            n196 = Build Array(w492) -> (w493:T6[])
            n197 = Unbundle By Name(w488) -> ("DevType"=w497:T5, "DevIndex"=w496:u32, "CanIndex"=w494:T4)
            n198 = call "VCI_Transmit.vi"("Buffer"=w493, "CANIndex"=w494, "DevIndex"=w496, "DevType"=w497) -> ()  [unwired: 1 in, 7 out]
          }
          event "看门狗_W": Value Change {
            w518 = u8 0 items=["数据帧", "遥控帧"]
            w510 = u32 138
            w519 = u8 0 items=["标准帧", "扩展帧"]
            n199 = event-data() -> ()  [unwired: 2 out]
            n200 = case shown="\"开启\", 默认" "看门狗" {
              tunnel: [w522 w527 w532] -> w507
              frame "开启", Default {
                n201 = Split Number(x=u16 52428) -> (hi(x)=w525:u8, lo(x)=w526:u8)
                n202 = Build Array(u8 2, w525, w526) -> (w522:u8[])
              }
              frame "喂狗" {
                n203 = Split Number(x=u16 43690) -> (hi(x)=w529:u8, lo(x)=w528:u8)
                n204 = Build Array(u8 2, w529, w528) -> (w527:u8[])
              }
              frame "关闭" {
                n205 = Split Number(x=u16 52394) -> (hi(x)=w534:u8, lo(x)=w533:u8)
                n206 = Build Array(u8 2, w534, w533) -> (w532:u8[])
              }
            }
            n207 = Bundle By Name(cluster=T6 {"ID"=0, "TimeStamp"=0, "TimeFlag"=0, "SendType"=0, "RemoteFlag"=0, "ExternFlag"=0, "DataLen"=0, "Data"=[], "Reserved"=[]} ("Send"), "ID"=w510, "RemoteFlag"=w518, "ExternFlag"=w519, "DataLen"=u8 3, "Data"=w507) -> (w517:T6)
            n208 = Build Array(w517) -> (w516:T6[])
            n209 = Unbundle By Name(w511) -> ("DevType"=w513:T5, "DevIndex"=w514:u32, "CanIndex"=w515:T4)
            n210 = call "VCI_Transmit.vi"("Buffer"=w516, "CANIndex"=w515, "DevIndex"=w514, "DevType"=w513) -> ()  [unwired: 1 in, 7 out]
          }
          event "模式_W": Value Change {
            w543 = u8 0 items=["数据帧", "遥控帧"]
            w542 = u8 0 items=["标准帧", "扩展帧"]
            # "地址"
            n211 = event-data() -> ()  [unwired: 2 out]
            n212 = property on="电机ID" class="CmbBox"() -> ("Value"=w552:string)  [unwired: 2 in, 2 out]
            n213 = Concatenate Strings("20 ", "模式") -> (w556:string)
            n214 = Scan From String(format string="%x" ("格式字符串"), input string=w552, default 1=u8 0) -> (output 1=w555:u8)  [unwired: 2 in, 3 out]
            n215 = property on="模式_回" class="CmbBox"("Value"="模式") -> ()  [unwired: 2 in, 2 out]
            n216 = call "Demo_MakeData.vi"("DataString"=w556) -> ("Data"=w539:u8[], "DataLen"=w547:u8)  [unwired: 9 out]
            n217 = Add(x=u32 16, y=w555) -> (x+y=w538:u32)
            n218 = Bundle By Name(cluster=T6 {"ID"=0, "TimeStamp"=0, "TimeFlag"=0, "SendType"=0, "RemoteFlag"=0, "ExternFlag"=0, "DataLen"=0, "Data"=[], "Reserved"=[]} ("Send"), "ID"=w538, "RemoteFlag"=w543, "ExternFlag"=w542, "DataLen"=w547, "Data"=w539) -> (w544:T6)
            n219 = Build Array(w544) -> (w545:T6[])
            n220 = Unbundle By Name(w541) -> ("DevType"=w549:T5, "DevIndex"=w548:u32, "CanIndex"=w546:T4)
            n221 = call "VCI_Transmit.vi"("Buffer"=w545, "CANIndex"=w546, "DevIndex"=w548, "DevType"=w549) -> ()  [unwired: 1 in, 7 out]
          }
          event "模式_R": Value Change {
            w576 = u8 0 items=["数据帧", "遥控帧"]
            w577 = u8 0 items=["标准帧", "扩展帧"]
            # "地址"
            n222 = event-data() -> ()  [unwired: 2 out]
            n223 = property on="电机ID" class="CmbBox"() -> ("Value"=w567:string)  [unwired: 2 in, 2 out]
            n224 = Scan From String(format string="%x" ("格式字符串"), input string=w567, default 1=u8 0) -> (output 1=w564:u8)  [unwired: 2 in, 3 out]
            n225 = call "Demo_MakeData.vi"("DataString"="20 ") -> ("Data"=w561:u8[], "DataLen"=w572:u8)  [unwired: 9 out]
            n226 = Add(x=u32 48, y=w564) -> (x+y=w560:u32)
            n227 = Bundle By Name(cluster=T6 {"ID"=0, "TimeStamp"=0, "TimeFlag"=0, "SendType"=0, "RemoteFlag"=0, "ExternFlag"=0, "DataLen"=0, "Data"=[], "Reserved"=[]} ("Send"), "ID"=w560, "RemoteFlag"=w576, "ExternFlag"=w577, "DataLen"=w572, "Data"=w561) -> (w575:T6)
            n228 = Build Array(w575) -> (w574:T6[])
            n229 = Unbundle By Name(w563) -> ("DevType"=w570:T5, "DevIndex"=w571:u32, "CanIndex"=w573:T4)
            n230 = call "VCI_Transmit.vi"("Buffer"=w574, "CANIndex"=w573, "DevIndex"=w571, "DevType"=w570) -> ()  [unwired: 1 in, 7 out]
          }
          event "设定位置_W": Value Change {
            w593 = u8 0 items=["数据帧", "遥控帧"]
            w592 = u8 0 items=["标准帧", "扩展帧"]
            # "索引地址"
            n231 = event-data() -> ()  [unwired: 2 out]
            n232 = property on="电机ID" class="CmbBox"() -> ("Value"=w601:string)  [unwired: 2 in, 2 out]
            n233 = Multiply ("乘")(x="设定位置", y=u16 256) -> (x*y=w585:i16)
            n234 = Scan From String(format string="%x" ("格式字符串"), input string=w601, default 1=u8 0) -> (output 1=w604:u8)  [unwired: 2 in, 3 out]
            n235 = Split Number(x=w585) -> (hi(x)=w584:u8, lo(x)=w583:u8)
            n236 = Add(x=u32 16, y=w604) -> (x+y=w581:u32)
            n237 = Build Array(u8 64, w584, w583) -> (w582:u8[])
            n238 = Bundle By Name(cluster=T6 {"ID"=0, "TimeStamp"=0, "TimeFlag"=0, "SendType"=0, "RemoteFlag"=0, "ExternFlag"=0, "DataLen"=0, "Data"=[], "Reserved"=[]} ("Send"), "ID"=w581, "RemoteFlag"=w593, "ExternFlag"=w592, "DataLen"=u8 3, "Data"=w582) -> (w594:T6)
            n239 = Build Array(w594) -> (w595:T6[])
            n240 = Unbundle By Name(w591) -> ("DevType"=w598:T5, "DevIndex"=w597:u32, "CanIndex"=w596:T4)
            n241 = call "VCI_Transmit.vi"("Buffer"=w595, "CANIndex"=w596, "DevIndex"=w597, "DevType"=w598) -> ()  [unwired: 1 in, 7 out]
          }
          event "设定速度_W": Value Change {
            w626 = u8 0 items=["数据帧", "遥控帧"]
            w627 = u8 0 items=["标准帧", "扩展帧"]
            # "索引地址"
            n242 = event-data() -> ()  [unwired: 2 out]
            n243 = property on="电机ID" class="CmbBox"() -> ("Value"=w618:string)  [unwired: 2 in, 2 out]
            n244 = Multiply ("乘")(x="设定速度", y=i16 1) -> (x*y=w611:i16)
            n245 = Scan From String(format string="%x" ("格式字符串"), input string=w618, default 1=u8 0) -> (output 1=w615:u8)  [unwired: 2 in, 3 out]
            n246 = Split Number(x=w611) -> (hi(x)=w610:u8, lo(x)=w609:u8)
            n247 = Add(x=u32 16, y=w615) -> (x+y=w607:u32)
            n248 = Build Array(u8 65, w610, w609) -> (w608:u8[])
            n249 = Bundle By Name(cluster=T6 {"ID"=0, "TimeStamp"=0, "TimeFlag"=0, "SendType"=0, "RemoteFlag"=0, "ExternFlag"=0, "DataLen"=0, "Data"=[], "Reserved"=[]} ("Send"), "ID"=w607, "RemoteFlag"=w626, "ExternFlag"=w627, "DataLen"=u8 3, "Data"=w608) -> (w625:T6)
            n250 = Build Array(w625) -> (w624:T6[])
            n251 = Unbundle By Name(w614) -> ("DevType"=w621:T5, "DevIndex"=w622:u32, "CanIndex"=w623:T4)
            n252 = call "VCI_Transmit.vi"("Buffer"=w624, "CANIndex"=w623, "DevIndex"=w622, "DevType"=w621) -> ()  [unwired: 1 in, 7 out]
          }
          event "设定电流_W": Value Change {
            w645 = u8 0 items=["数据帧", "遥控帧"]
            w644 = u8 0 items=["标准帧", "扩展帧"]
            # "索引地址"
            n253 = event-data() -> ()  [unwired: 2 out]
            n254 = property on="电机ID" class="CmbBox"() -> ("Value"=w653:string)  [unwired: 2 in, 2 out]
            n255 = Multiply ("乘")(x="设定电流", y=i16 256) -> (x*y=w637:i16)
            n256 = Scan From String(format string="%x" ("格式字符串"), input string=w653, default 1=u8 0) -> (output 1=w656:u8)  [unwired: 2 in, 3 out]
            n257 = Split Number(x=w637) -> (hi(x)=w636:u8, lo(x)=w635:u8)
            n258 = Add(x=u32 16, y=w656) -> (x+y=w633:u32)
            n259 = Build Array(u8 66, w636, w635) -> (w634:u8[])
            n260 = Bundle By Name(cluster=T6 {"ID"=0, "TimeStamp"=0, "TimeFlag"=0, "SendType"=0, "RemoteFlag"=0, "ExternFlag"=0, "DataLen"=0, "Data"=[], "Reserved"=[]} ("Send"), "ID"=w633, "RemoteFlag"=w645, "ExternFlag"=w644, "DataLen"=u8 3, "Data"=w634) -> (w646:T6)
            n261 = Build Array(w646) -> (w647:T6[])
            n262 = Unbundle By Name(w640) -> ("DevType"=w650:T5, "DevIndex"=w649:u32, "CanIndex"=w648:T4)
            n263 = call "VCI_Transmit.vi"("Buffer"=w647, "CANIndex"=w648, "DevIndex"=w649, "DevType"=w650) -> ()  [unwired: 1 in, 7 out]
          }
          event "Direction_W": Value Change {
            w676 = u8 0 items=["数据帧", "遥控帧"]
            w677 = u8 0 items=["标准帧", "扩展帧"]
            # "索引地址"
            n264 = event-data() -> ()  [unwired: 2 out]
            n265 = property on="电机ID" class="CmbBox"() -> ("Value"=w668:string)  [unwired: 2 in, 2 out]
            n266 = Scan From String(format string="%x" ("格式字符串"), input string=w668, default 1=u8 0) -> (output 1=w665:u8)  [unwired: 2 in, 3 out]
            n267 = Add(x=u32 16, y=w665) -> (x+y=w661:u32)
            n268 = Build Array(u8 106, "方向") -> (w662:u16[])
            n269 = Bundle By Name(cluster=T6 {"ID"=0, "TimeStamp"=0, "TimeFlag"=0, "SendType"=0, "RemoteFlag"=0, "ExternFlag"=0, "DataLen"=0, "Data"=[], "Reserved"=[]} ("Send"), "ID"=w661, "RemoteFlag"=w676, "ExternFlag"=w677, "DataLen"=u8 2, "Data"=w662) -> (w675:T6)
            n270 = Build Array(w675) -> (w674:T6[])
            n271 = Unbundle By Name(w664) -> ("DevType"=w671:T5, "DevIndex"=w672:u32, "CanIndex"=w673:T4)
            n272 = call "VCI_Transmit.vi"("Buffer"=w674, "CANIndex"=w673, "DevIndex"=w672, "DevType"=w671) -> ()  [unwired: 1 in, 7 out]
          }
          event "I_EN_W": Value Change {
            w689 = u8 0 items=["数据帧", "遥控帧"]
            w688 = u8 0 items=["标准帧", "扩展帧"]
            # "索引地址"
            n273 = event-data() -> ()  [unwired: 2 out]
            n274 = property on="电机ID" class="CmbBox"() -> ("Value"=w697:string)  [unwired: 2 in, 2 out]
            n275 = Scan From String(format string="%x" ("格式字符串"), input string=w697, default 1=u8 0) -> (output 1=w700:u8)  [unwired: 2 in, 3 out]
            n276 = Add(x=u32 16, y=w700) -> (x+y=w682:u32)
            n277 = Build Array(u8 104, "电流诊断使能") -> (w683:u8[])
            n278 = Bundle By Name(cluster=T6 {"ID"=0, "TimeStamp"=0, "TimeFlag"=0, "SendType"=0, "RemoteFlag"=0, "ExternFlag"=0, "DataLen"=0, "Data"=[], "Reserved"=[]} ("Send"), "ID"=w682, "RemoteFlag"=w689, "ExternFlag"=w688, "DataLen"=u8 2, "Data"=w683) -> (w690:T6)
            n279 = Build Array(w690) -> (w691:T6[])
            n280 = Unbundle By Name(w685) -> ("DevType"=w694:T5, "DevIndex"=w693:u32, "CanIndex"=w692:T4)
            n281 = call "VCI_Transmit.vi"("Buffer"=w691, "CANIndex"=w692, "DevIndex"=w693, "DevType"=w694) -> ()  [unwired: 1 in, 7 out]
          }
          event "W_EN_W": Value Change {
            w711 = u8 0 items=["数据帧", "遥控帧"]
            w710 = u8 0 items=["标准帧", "扩展帧"]
            # "索引地址"
            n282 = event-data() -> ()  [unwired: 2 out]
            n283 = property on="电机ID" class="CmbBox"() -> ("Value"=w719:string)  [unwired: 2 in, 2 out]
            n284 = Scan From String(format string="%x" ("格式字符串"), input string=w719, default 1=u8 0) -> (output 1=w722:u8)  [unwired: 2 in, 3 out]
            n285 = Add(x=u32 16, y=w722) -> (x+y=w704:u32)
            n286 = Build Array(u8 105, "过载诊断使能") -> (w705:u8[])
            n287 = Bundle By Name(cluster=T6 {"ID"=0, "TimeStamp"=0, "TimeFlag"=0, "SendType"=0, "RemoteFlag"=0, "ExternFlag"=0, "DataLen"=0, "Data"=[], "Reserved"=[]} ("Send"), "ID"=w704, "RemoteFlag"=w711, "ExternFlag"=w710, "DataLen"=u8 2, "Data"=w705) -> (w712:T6)
            n288 = Build Array(w712) -> (w713:T6[])
            n289 = Unbundle By Name(w707) -> ("DevType"=w716:T5, "DevIndex"=w715:u32, "CanIndex"=w714:T4)
            n290 = call "VCI_Transmit.vi"("Buffer"=w713, "CANIndex"=w714, "DevIndex"=w715, "DevType"=w716) -> ()  [unwired: 1 in, 7 out]
          }
          event "速度环KI_W": Value Change {
            w741 = u8 0 items=["数据帧", "遥控帧"]
            w742 = u8 0 items=["标准帧", "扩展帧"]
            # "索引地址"
            n291 = event-data() -> ()  [unwired: 2 out]
            n292 = property on="电机ID" class="CmbBox"() -> ("Value"=w733:string)  [unwired: 2 in, 2 out]
            n293 = Multiply ("乘")(x="速度环KI", y=u16 256) -> (x*y=w746:u16)
            n294 = Scan From String(format string="%x" ("格式字符串"), input string=w733, default 1=u8 0) -> (output 1=w730:u8)  [unwired: 2 in, 3 out]
            n295 = Split Number(x=w746) -> (hi(x)=w747:u8, lo(x)=w748:u8)
            n296 = Add(x=u32 16, y=w730) -> (x+y=w725:u32)
            n297 = Build Array(u8 84, w747, w748) -> (w726:u8[])
            n298 = Bundle By Name(cluster=T6 {"ID"=0, "TimeStamp"=0, "TimeFlag"=0, "SendType"=0, "RemoteFlag"=0, "ExternFlag"=0, "DataLen"=0, "Data"=[], "Reserved"=[]} ("Send"), "ID"=w725, "RemoteFlag"=w741, "ExternFlag"=w742, "DataLen"=u8 3, "Data"=w726) -> (w740:T6)
            n299 = Build Array(w740) -> (w739:T6[])
            n300 = Unbundle By Name(w729) -> ("DevType"=w736:T5, "DevIndex"=w737:u32, "CanIndex"=w738:T4)
            n301 = call "VCI_Transmit.vi"("Buffer"=w739, "CANIndex"=w738, "DevIndex"=w737, "DevType"=w736) -> ()  [unwired: 1 in, 7 out]
          }
          event "加速度_W": Value Change {
            w763 = u8 0 items=["数据帧", "遥控帧"]
            w762 = u8 0 items=["标准帧", "扩展帧"]
            # "索引地址"
            n302 = event-data() -> ()  [unwired: 2 out]
            n303 = property on="电机ID" class="CmbBox"() -> ("Value"=w771:string)  [unwired: 2 in, 2 out]
            n304 = Multiply ("乘")(x="加速度", y=u16 8) -> (x*y=w758:u16)
            n305 = Scan From String(format string="%x" ("格式字符串"), input string=w771, default 1=u8 0) -> (output 1=w774:u8)  [unwired: 2 in, 3 out]
            n306 = Split Number(x=w758) -> (hi(x)=w757:u8, lo(x)=w756:u8)
            n307 = Add(x=u32 16, y=w774) -> (x+y=w751:u32)
            n308 = Build Array(u8 85, w757, w756) -> (w752:u8[])
            n309 = Bundle By Name(cluster=T6 {"ID"=0, "TimeStamp"=0, "TimeFlag"=0, "SendType"=0, "RemoteFlag"=0, "ExternFlag"=0, "DataLen"=0, "Data"=[], "Reserved"=[]} ("Send"), "ID"=w751, "RemoteFlag"=w763, "ExternFlag"=w762, "DataLen"=u8 3, "Data"=w752) -> (w764:T6)
            n310 = Build Array(w764) -> (w765:T6[])
            n311 = Unbundle By Name(w755) -> ("DevType"=w768:T5, "DevIndex"=w767:u32, "CanIndex"=w766:T4)
            n312 = call "VCI_Transmit.vi"("Buffer"=w765, "CANIndex"=w766, "DevIndex"=w767, "DevType"=w768) -> ()  [unwired: 1 in, 7 out]
          }
          event "减速度_W": Value Change {
            w793 = u8 0 items=["数据帧", "遥控帧"]
            w794 = u8 0 items=["标准帧", "扩展帧"]
            # "索引地址"
            n313 = event-data() -> ()  [unwired: 2 out]
            n314 = property on="电机ID" class="CmbBox"() -> ("Value"=w785:string)  [unwired: 2 in, 2 out]
            n315 = Multiply ("乘")(x="减速度", y=u16 8) -> (x*y=w798:u16)
            n316 = Scan From String(format string="%x" ("格式字符串"), input string=w785, default 1=u8 0) -> (output 1=w782:u8)  [unwired: 2 in, 3 out]
            n317 = Split Number(x=w798) -> (hi(x)=w799:u8, lo(x)=w800:u8)
            n318 = Add(x=u32 16, y=w782) -> (x+y=w778:u32)
            n319 = Build Array(u8 86, w799, w800) -> (w779:u8[])
            n320 = Bundle By Name(cluster=T6 {"ID"=0, "TimeStamp"=0, "TimeFlag"=0, "SendType"=0, "RemoteFlag"=0, "ExternFlag"=0, "DataLen"=0, "Data"=[], "Reserved"=[]} ("Send"), "ID"=w778, "RemoteFlag"=w793, "ExternFlag"=w794, "DataLen"=u8 3, "Data"=w779) -> (w792:T6)
            n321 = Build Array(w792) -> (w791:T6[])
            n322 = Unbundle By Name(w781) -> ("DevType"=w788:T5, "DevIndex"=w789:u32, "CanIndex"=w790:T4)
            n323 = call "VCI_Transmit.vi"("Buffer"=w791, "CANIndex"=w790, "DevIndex"=w789, "DevType"=w788) -> ()  [unwired: 1 in, 7 out]
          }
          event "T1_W": Value Change {
            w813 = u8 0 items=["数据帧", "遥控帧"]
            w812 = u8 0 items=["标准帧", "扩展帧"]
            # "索引地址"
            n324 = event-data() -> ()  [unwired: 2 out]
            n325 = property on="电机ID" class="CmbBox"() -> ("Value"=w821:string)  [unwired: 2 in, 2 out]
            n326 = Scan From String(format string="%x" ("格式字符串"), input string=w821, default 1=u8 0) -> (output 1=w824:u8)  [unwired: 2 in, 3 out]
            n327 = Split Number(x="T1") -> (hi(x)=w809:u8, lo(x)=w808:u8)
            n328 = Add(x=u32 16, y=w824) -> (x+y=w803:u32)
            n329 = Build Array(u8 100, w809, w808) -> (w804:u8[])
            n330 = Bundle By Name(cluster=T6 {"ID"=0, "TimeStamp"=0, "TimeFlag"=0, "SendType"=0, "RemoteFlag"=0, "ExternFlag"=0, "DataLen"=0, "Data"=[], "Reserved"=[]} ("Send"), "ID"=w803, "RemoteFlag"=w813, "ExternFlag"=w812, "DataLen"=u8 3, "Data"=w804) -> (w814:T6)
            n331 = Build Array(w814) -> (w815:T6[])
            n332 = Unbundle By Name(w807) -> ("DevType"=w818:T5, "DevIndex"=w817:u32, "CanIndex"=w816:T4)
            n333 = call "VCI_Transmit.vi"("Buffer"=w815, "CANIndex"=w816, "DevIndex"=w817, "DevType"=w818) -> ()  [unwired: 1 in, 7 out]
          }
          event "T2_W": Value Change {
            w837 = u8 0 items=["数据帧", "遥控帧"]
            w836 = u8 0 items=["标准帧", "扩展帧"]
            # "索引地址"
            n334 = event-data() -> ()  [unwired: 2 out]
            n335 = property on="电机ID" class="CmbBox"() -> ("Value"=w845:string)  [unwired: 2 in, 2 out]
            n336 = Scan From String(format string="%x" ("格式字符串"), input string=w845, default 1=u8 0) -> (output 1=w848:u8)  [unwired: 2 in, 3 out]
            n337 = Split Number(x="T2") -> (hi(x)=w833:u8, lo(x)=w832:u8)
            n338 = Add(x=u32 16, y=w848) -> (x+y=w827:u32)
            n339 = Build Array(u8 101, w833, w832) -> (w828:u8[])
            n340 = Bundle By Name(cluster=T6 {"ID"=0, "TimeStamp"=0, "TimeFlag"=0, "SendType"=0, "RemoteFlag"=0, "ExternFlag"=0, "DataLen"=0, "Data"=[], "Reserved"=[]} ("Send"), "ID"=w827, "RemoteFlag"=w837, "ExternFlag"=w836, "DataLen"=u8 3, "Data"=w828) -> (w838:T6)
            n341 = Build Array(w838) -> (w839:T6[])
            n342 = Unbundle By Name(w831) -> ("DevType"=w842:T5, "DevIndex"=w841:u32, "CanIndex"=w840:T4)
            n343 = call "VCI_Transmit.vi"("Buffer"=w839, "CANIndex"=w840, "DevIndex"=w841, "DevType"=w842) -> ()  [unwired: 1 in, 7 out]
          }
          event "T3_W": Value Change {
            w861 = u8 0 items=["数据帧", "遥控帧"]
            w860 = u8 0 items=["标准帧", "扩展帧"]
            # "索引地址"
            n344 = event-data() -> ()  [unwired: 2 out]
            n345 = property on="电机ID" class="CmbBox"() -> ("Value"=w869:string)  [unwired: 2 in, 2 out]
            n346 = Scan From String(format string="%x" ("格式字符串"), input string=w869, default 1=u8 0) -> (output 1=w872:u8)  [unwired: 2 in, 3 out]
            n347 = Split Number(x="T3") -> (hi(x)=w857:u8, lo(x)=w856:u8)
            n348 = Add(x=u32 16, y=w872) -> (x+y=w851:u32)
            n349 = Build Array(u8 102, w857, w856) -> (w852:u8[])
            n350 = Bundle By Name(cluster=T6 {"ID"=0, "TimeStamp"=0, "TimeFlag"=0, "SendType"=0, "RemoteFlag"=0, "ExternFlag"=0, "DataLen"=0, "Data"=[], "Reserved"=[]} ("Send"), "ID"=w851, "RemoteFlag"=w861, "ExternFlag"=w860, "DataLen"=u8 3, "Data"=w852) -> (w862:T6)
            n351 = Build Array(w862) -> (w863:T6[])
            n352 = Unbundle By Name(w855) -> ("DevType"=w866:T5, "DevIndex"=w865:u32, "CanIndex"=w864:T4)
            n353 = call "VCI_Transmit.vi"("Buffer"=w863, "CANIndex"=w864, "DevIndex"=w865, "DevType"=w866) -> ()  [unwired: 1 in, 7 out]
          }
          event "T4_W": Value Change {
            w891 = u8 0 items=["数据帧", "遥控帧"]
            w892 = u8 0 items=["标准帧", "扩展帧"]
            # "索引地址"
            n354 = event-data() -> ()  [unwired: 2 out]
            n355 = property on="电机ID" class="CmbBox"() -> ("Value"=w883:string)  [unwired: 2 in, 2 out]
            n356 = Scan From String(format string="%x" ("格式字符串"), input string=w883, default 1=u8 0) -> (output 1=w880:u8)  [unwired: 2 in, 3 out]
            n357 = Add(x=u32 16, y=w880) -> (x+y=w878:u32)
            n358 = Split Number(x="T4") -> (hi(x)=w895:u8, lo(x)=w896:u8)
            n359 = Build Array(u8 103, w895, w896) -> (w877:u8[])
            n360 = Bundle By Name(cluster=T6 {"ID"=0, "TimeStamp"=0, "TimeFlag"=0, "SendType"=0, "RemoteFlag"=0, "ExternFlag"=0, "DataLen"=0, "Data"=[], "Reserved"=[]} ("Send"), "ID"=w878, "RemoteFlag"=w891, "ExternFlag"=w892, "DataLen"=u8 3, "Data"=w877) -> (w890:T6)
            n361 = Build Array(w890) -> (w889:T6[])
            n362 = Unbundle By Name(w879) -> ("DevType"=w886:T5, "DevIndex"=w887:u32, "CanIndex"=w888:T4)
            n363 = call "VCI_Transmit.vi"("Buffer"=w889, "CANIndex"=w888, "DevIndex"=w887, "DevType"=w886) -> ()  [unwired: 1 in, 7 out]
          }
          event "DATA_SAVE_W": Value Change {
            w915 = u8 0 items=["数据帧", "遥控帧"]
            w916 = u8 0 items=["标准帧", "扩展帧"]
            # "地址"
            n364 = event-data() -> ()  [unwired: 2 out]
            n365 = property on="电机ID" class="CmbBox"() -> ("Value"=w906:string)  [unwired: 2 in, 2 out]
            n366 = Scan From String(format string="%x" ("格式字符串"), input string=w906, default 1=u8 0) -> (output 1=w903:u8)  [unwired: 2 in, 3 out]
            n367 = call "Demo_MakeData.vi"("DataString"="50") -> ("Data"=w900:u8[], "DataLen"=w911:u8)  [unwired: 9 out]
            n368 = Add(x=u32 16, y=w903) -> (x+y=w899:u32)
            n369 = Bundle By Name(cluster=T6 {"ID"=0, "TimeStamp"=0, "TimeFlag"=0, "SendType"=0, "RemoteFlag"=0, "ExternFlag"=0, "DataLen"=0, "Data"=[], "Reserved"=[]} ("Send"), "ID"=w899, "RemoteFlag"=w915, "ExternFlag"=w916, "DataLen"=w911, "Data"=w900) -> (w914:T6)
            n370 = Build Array(w914) -> (w913:T6[])
            n371 = Unbundle By Name(w902) -> ("DevType"=w909:T5, "DevIndex"=w910:u32, "CanIndex"=w912:T4)
            n372 = call "VCI_Transmit.vi"("Buffer"=w913, "CANIndex"=w912, "DevIndex"=w910, "DevType"=w909) -> ()  [unwired: 1 in, 7 out]
          }
          event "设定位置_R": Value Change {
            w926 = u8 0 items=["数据帧", "遥控帧"]
            w925 = u8 0 items=["标准帧", "扩展帧"]
            # "地址"
            n373 = event-data() -> ()  [unwired: 2 out]
            n374 = property on="电机ID" class="CmbBox"() -> ("Value"=w935:string)  [unwired: 2 in, 2 out]
            n375 = Scan From String(format string="%x" ("格式字符串"), input string=w935, default 1=u8 0) -> (output 1=w938:u8)  [unwired: 2 in, 3 out]
            n376 = call "Demo_MakeData.vi"("DataString"="40 ") -> ("Data"=w921:u8[], "DataLen"=w930:u8)  [unwired: 9 out]
            n377 = Add(x=u32 48, y=w938) -> (x+y=w920:u32)
            n378 = Bundle By Name(cluster=T6 {"ID"=0, "TimeStamp"=0, "TimeFlag"=0, "SendType"=0, "RemoteFlag"=0, "ExternFlag"=0, "DataLen"=0, "Data"=[], "Reserved"=[]} ("Send"), "ID"=w920, "RemoteFlag"=w926, "ExternFlag"=w925, "DataLen"=w930, "Data"=w921) -> (w927:T6)
            n379 = Build Array(w927) -> (w928:T6[])
            n380 = Unbundle By Name(w923) -> ("DevType"=w932:T5, "DevIndex"=w931:u32, "CanIndex"=w929:T4)
            n381 = call "VCI_Transmit.vi"("Buffer"=w928, "CANIndex"=w929, "DevIndex"=w931, "DevType"=w932) -> ()  [unwired: 1 in, 7 out]
          }
          event "设定速度_R": Value Change {
            w957 = u8 0 items=["数据帧", "遥控帧"]
            w958 = u8 0 items=["标准帧", "扩展帧"]
            # "地址"
            n382 = event-data() -> ()  [unwired: 2 out]
            n383 = property on="电机ID" class="CmbBox"() -> ("Value"=w948:string)  [unwired: 2 in, 2 out]
            n384 = Scan From String(format string="%x" ("格式字符串"), input string=w948, default 1=u8 0) -> (output 1=w945:u8)  [unwired: 2 in, 3 out]
            n385 = call "Demo_MakeData.vi"("DataString"="41 ") -> ("Data"=w942:u8[], "DataLen"=w953:u8)  [unwired: 9 out]
            n386 = Add(x=u32 48, y=w945) -> (x+y=w941:u32)
            n387 = Bundle By Name(cluster=T6 {"ID"=0, "TimeStamp"=0, "TimeFlag"=0, "SendType"=0, "RemoteFlag"=0, "ExternFlag"=0, "DataLen"=0, "Data"=[], "Reserved"=[]} ("Send"), "ID"=w941, "RemoteFlag"=w957, "ExternFlag"=w958, "DataLen"=w953, "Data"=w942) -> (w956:T6)
            n388 = Build Array(w956) -> (w955:T6[])
            n389 = Unbundle By Name(w944) -> ("DevType"=w951:T5, "DevIndex"=w952:u32, "CanIndex"=w954:T4)
            n390 = call "VCI_Transmit.vi"("Buffer"=w955, "CANIndex"=w954, "DevIndex"=w952, "DevType"=w951) -> ()  [unwired: 1 in, 7 out]
          }
          event "设定电流_R": Value Change {
            w978 = u8 0 items=["数据帧", "遥控帧"]
            w979 = u8 0 items=["标准帧", "扩展帧"]
            # "地址"
            n391 = event-data() -> ()  [unwired: 2 out]
            n392 = property on="电机ID" class="CmbBox"() -> ("Value"=w969:string)  [unwired: 2 in, 2 out]
            n393 = Scan From String(format string="%x" ("格式字符串"), input string=w969, default 1=u8 0) -> (output 1=w966:u8)  [unwired: 2 in, 3 out]
            n394 = call "Demo_MakeData.vi"("DataString"="42 ") -> ("Data"=w963:u8[], "DataLen"=w974:u8)  [unwired: 9 out]
            n395 = Add(x=u32 48, y=w966) -> (x+y=w962:u32)
            n396 = Bundle By Name(cluster=T6 {"ID"=0, "TimeStamp"=0, "TimeFlag"=0, "SendType"=0, "RemoteFlag"=0, "ExternFlag"=0, "DataLen"=0, "Data"=[], "Reserved"=[]} ("Send"), "ID"=w962, "RemoteFlag"=w978, "ExternFlag"=w979, "DataLen"=w974, "Data"=w963) -> (w977:T6)
            n397 = Build Array(w977) -> (w976:T6[])
            n398 = Unbundle By Name(w965) -> ("DevType"=w972:T5, "DevIndex"=w973:u32, "CanIndex"=w975:T4)
            n399 = call "VCI_Transmit.vi"("Buffer"=w976, "CANIndex"=w975, "DevIndex"=w973, "DevType"=w972) -> ()  [unwired: 1 in, 7 out]
          }
          event "Direction_R": Value Change {
            w999 = u8 0 items=["数据帧", "遥控帧"]
            w1000 = u8 0 items=["标准帧", "扩展帧"]
            # "地址"
            n400 = event-data() -> ()  [unwired: 2 out]
            n401 = property on="电机ID" class="CmbBox"() -> ("Value"=w990:string)  [unwired: 2 in, 2 out]
            n402 = Scan From String(format string="%x" ("格式字符串"), input string=w990, default 1=u8 0) -> (output 1=w987:u8)  [unwired: 2 in, 3 out]
            n403 = call "Demo_MakeData.vi"("DataString"="6A ") -> ("Data"=w984:u8[], "DataLen"=w995:u8)  [unwired: 9 out]
            n404 = Add(x=u32 48, y=w987) -> (x+y=w983:u32)
            n405 = Bundle By Name(cluster=T6 {"ID"=0, "TimeStamp"=0, "TimeFlag"=0, "SendType"=0, "RemoteFlag"=0, "ExternFlag"=0, "DataLen"=0, "Data"=[], "Reserved"=[]} ("Send"), "ID"=w983, "RemoteFlag"=w999, "ExternFlag"=w1000, "DataLen"=w995, "Data"=w984) -> (w998:T6)
            n406 = Build Array(w998) -> (w997:T6[])
            n407 = Unbundle By Name(w986) -> ("DevType"=w993:T5, "DevIndex"=w994:u32, "CanIndex"=w996:T4)
            n408 = call "VCI_Transmit.vi"("Buffer"=w997, "CANIndex"=w996, "DevIndex"=w994, "DevType"=w993) -> ()  [unwired: 1 in, 7 out]
          }
          event "I_EN_R": Value Change {
            w1020 = u8 0 items=["数据帧", "遥控帧"]
            w1021 = u8 0 items=["标准帧", "扩展帧"]
            # "地址"
            n409 = event-data() -> ()  [unwired: 2 out]
            n410 = property on="电机ID" class="CmbBox"() -> ("Value"=w1011:string)  [unwired: 2 in, 2 out]
            n411 = Scan From String(format string="%x" ("格式字符串"), input string=w1011, default 1=u8 0) -> (output 1=w1008:u8)  [unwired: 2 in, 3 out]
            n412 = call "Demo_MakeData.vi"("DataString"="68 ") -> ("Data"=w1005:u8[], "DataLen"=w1016:u8)  [unwired: 9 out]
            n413 = Add(x=u32 48, y=w1008) -> (x+y=w1004:u32)
            n414 = Bundle By Name(cluster=T6 {"ID"=0, "TimeStamp"=0, "TimeFlag"=0, "SendType"=0, "RemoteFlag"=0, "ExternFlag"=0, "DataLen"=0, "Data"=[], "Reserved"=[]} ("Send"), "ID"=w1004, "RemoteFlag"=w1020, "ExternFlag"=w1021, "DataLen"=w1016, "Data"=w1005) -> (w1019:T6)
            n415 = Build Array(w1019) -> (w1018:T6[])
            n416 = Unbundle By Name(w1007) -> ("DevType"=w1014:T5, "DevIndex"=w1015:u32, "CanIndex"=w1017:T4)
            n417 = call "VCI_Transmit.vi"("Buffer"=w1018, "CANIndex"=w1017, "DevIndex"=w1015, "DevType"=w1014) -> ()  [unwired: 1 in, 7 out]
          }
          event "W_EN_R": Value Change {
            w1032 = u8 0 items=["数据帧", "遥控帧"]
            w1031 = u8 0 items=["标准帧", "扩展帧"]
            # "地址"
            n418 = event-data() -> ()  [unwired: 2 out]
            n419 = property on="电机ID" class="CmbBox"() -> ("Value"=w1040:string)  [unwired: 2 in, 2 out]
            n420 = Scan From String(format string="%x" ("格式字符串"), input string=w1040, default 1=u8 0) -> (output 1=w1043:u8)  [unwired: 2 in, 3 out]
            n421 = call "Demo_MakeData.vi"("DataString"="69 ") -> ("Data"=w1027:u8[], "DataLen"=w1025:u8)  [unwired: 9 out]
            n422 = Add(x=u32 48, y=w1043) -> (x+y=w1026:u32)
            n423 = Bundle By Name(cluster=T6 {"ID"=0, "TimeStamp"=0, "TimeFlag"=0, "SendType"=0, "RemoteFlag"=0, "ExternFlag"=0, "DataLen"=0, "Data"=[], "Reserved"=[]} ("Send"), "ID"=w1026, "RemoteFlag"=w1032, "ExternFlag"=w1031, "DataLen"=w1025, "Data"=w1027) -> (w1033:T6)
            n424 = Build Array(w1033) -> (w1034:T6[])
            n425 = Unbundle By Name(w1029) -> ("DevType"=w1037:T5, "DevIndex"=w1036:u32, "CanIndex"=w1035:T4)
            n426 = call "VCI_Transmit.vi"("Buffer"=w1034, "CANIndex"=w1035, "DevIndex"=w1036, "DevType"=w1037) -> ()  [unwired: 1 in, 7 out]
          }
          event "速度环KI_R": Value Change {
            w1052 = u8 0 items=["数据帧", "遥控帧"]
            w1051 = u8 0 items=["标准帧", "扩展帧"]
            # "地址"
            n427 = event-data() -> ()  [unwired: 2 out]
            n428 = property on="电机ID" class="CmbBox"() -> ("Value"=w1061:string)  [unwired: 2 in, 2 out]
            n429 = Scan From String(format string="%x" ("格式字符串"), input string=w1061, default 1=u8 0) -> (output 1=w1064:u8)  [unwired: 2 in, 3 out]
            n430 = call "Demo_MakeData.vi"("DataString"="54 ") -> ("Data"=w1047:u8[], "DataLen"=w1056:u8)  [unwired: 9 out]
            n431 = Add(x=u32 48, y=w1064) -> (x+y=w1046:u32)
            n432 = Bundle By Name(cluster=T6 {"ID"=0, "TimeStamp"=0, "TimeFlag"=0, "SendType"=0, "RemoteFlag"=0, "ExternFlag"=0, "DataLen"=0, "Data"=[], "Reserved"=[]} ("Send"), "ID"=w1046, "RemoteFlag"=w1052, "ExternFlag"=w1051, "DataLen"=w1056, "Data"=w1047) -> (w1053:T6)
            n433 = Build Array(w1053) -> (w1054:T6[])
            n434 = Unbundle By Name(w1049) -> ("DevType"=w1058:T5, "DevIndex"=w1057:u32, "CanIndex"=w1055:T4)
            n435 = call "VCI_Transmit.vi"("Buffer"=w1054, "CANIndex"=w1055, "DevIndex"=w1057, "DevType"=w1058) -> ()  [unwired: 1 in, 7 out]
          }
          event "加速度_R": Value Change {
            w1083 = u8 0 items=["数据帧", "遥控帧"]
            w1084 = u8 0 items=["标准帧", "扩展帧"]
            # "地址"
            n436 = event-data() -> ()  [unwired: 2 out]
            n437 = property on="电机ID" class="CmbBox"() -> ("Value"=w1074:string)  [unwired: 2 in, 2 out]
            n438 = Scan From String(format string="%x" ("格式字符串"), input string=w1074, default 1=u8 0) -> (output 1=w1071:u8)  [unwired: 2 in, 3 out]
            n439 = call "Demo_MakeData.vi"("DataString"="55") -> ("Data"=w1068:u8[], "DataLen"=w1079:u8)  [unwired: 9 out]
            n440 = Add(x=u32 48, y=w1071) -> (x+y=w1067:u32)
            n441 = Bundle By Name(cluster=T6 {"ID"=0, "TimeStamp"=0, "TimeFlag"=0, "SendType"=0, "RemoteFlag"=0, "ExternFlag"=0, "DataLen"=0, "Data"=[], "Reserved"=[]} ("Send"), "ID"=w1067, "RemoteFlag"=w1083, "ExternFlag"=w1084, "DataLen"=w1079, "Data"=w1068) -> (w1082:T6)
            n442 = Build Array(w1082) -> (w1081:T6[])
            n443 = Unbundle By Name(w1070) -> ("DevType"=w1077:T5, "DevIndex"=w1078:u32, "CanIndex"=w1080:T4)
            n444 = call "VCI_Transmit.vi"("Buffer"=w1081, "CANIndex"=w1080, "DevIndex"=w1078, "DevType"=w1077) -> ()  [unwired: 1 in, 7 out]
          }
          event "减速度_R": Value Change {
            w1094 = u8 0 items=["数据帧", "遥控帧"]
            w1093 = u8 0 items=["标准帧", "扩展帧"]
            # "地址"
            n445 = event-data() -> ()  [unwired: 2 out]
            n446 = property on="电机ID" class="CmbBox"() -> ("Value"=w1103:string)  [unwired: 2 in, 2 out]
            n447 = Scan From String(format string="%x" ("格式字符串"), input string=w1103, default 1=u8 0) -> (output 1=w1106:u8)  [unwired: 2 in, 3 out]
            n448 = call "Demo_MakeData.vi"("DataString"="56") -> ("Data"=w1089:u8[], "DataLen"=w1098:u8)  [unwired: 9 out]
            n449 = Add(x=u32 48, y=w1106) -> (x+y=w1090:u32)
            n450 = Bundle By Name(cluster=T6 {"ID"=0, "TimeStamp"=0, "TimeFlag"=0, "SendType"=0, "RemoteFlag"=0, "ExternFlag"=0, "DataLen"=0, "Data"=[], "Reserved"=[]} ("Send"), "ID"=w1090, "RemoteFlag"=w1094, "ExternFlag"=w1093, "DataLen"=w1098, "Data"=w1089) -> (w1095:T6)
            n451 = Build Array(w1095) -> (w1096:T6[])
            n452 = Unbundle By Name(w1091) -> ("DevType"=w1100:T5, "DevIndex"=w1099:u32, "CanIndex"=w1097:T4)
            n453 = call "VCI_Transmit.vi"("Buffer"=w1096, "CANIndex"=w1097, "DevIndex"=w1099, "DevType"=w1100) -> ()  [unwired: 1 in, 7 out]
          }
          event "T1_R": Value Change {
            w1115 = u8 0 items=["数据帧", "遥控帧"]
            w1114 = u8 0 items=["标准帧", "扩展帧"]
            # "地址"
            n454 = event-data() -> ()  [unwired: 2 out]
            n455 = property on="电机ID" class="CmbBox"() -> ("Value"=w1124:string)  [unwired: 2 in, 2 out]
            n456 = Scan From String(format string="%x" ("格式字符串"), input string=w1124, default 1=u8 0) -> (output 1=w1127:u8)  [unwired: 2 in, 3 out]
            n457 = call "Demo_MakeData.vi"("DataString"="64") -> ("Data"=w1110:u8[], "DataLen"=w1119:u8)  [unwired: 9 out]
            n458 = Add(x=u32 48, y=w1127) -> (x+y=w1109:u32)
            n459 = Bundle By Name(cluster=T6 {"ID"=0, "TimeStamp"=0, "TimeFlag"=0, "SendType"=0, "RemoteFlag"=0, "ExternFlag"=0, "DataLen"=0, "Data"=[], "Reserved"=[]} ("Send"), "ID"=w1109, "RemoteFlag"=w1115, "ExternFlag"=w1114, "DataLen"=w1119, "Data"=w1110) -> (w1116:T6)
            n460 = Build Array(w1116) -> (w1117:T6[])
            n461 = Unbundle By Name(w1112) -> ("DevType"=w1121:T5, "DevIndex"=w1120:u32, "CanIndex"=w1118:T4)
            n462 = call "VCI_Transmit.vi"("Buffer"=w1117, "CANIndex"=w1118, "DevIndex"=w1120, "DevType"=w1121) -> ()  [unwired: 1 in, 7 out]
          }
          event "T2_R": Value Change {
            w1136 = u8 0 items=["数据帧", "遥控帧"]
            w1135 = u8 0 items=["标准帧", "扩展帧"]
            # "地址"
            n463 = event-data() -> ()  [unwired: 2 out]
            n464 = property on="电机ID" class="CmbBox"() -> ("Value"=w1145:string)  [unwired: 2 in, 2 out]
            n465 = Scan From String(format string="%x" ("格式字符串"), input string=w1145, default 1=u8 0) -> (output 1=w1148:u8)  [unwired: 2 in, 3 out]
            n466 = call "Demo_MakeData.vi"("DataString"="65") -> ("Data"=w1131:u8[], "DataLen"=w1140:u8)  [unwired: 9 out]
            n467 = Add(x=u32 48, y=w1148) -> (x+y=w1130:u32)
            n468 = Bundle By Name(cluster=T6 {"ID"=0, "TimeStamp"=0, "TimeFlag"=0, "SendType"=0, "RemoteFlag"=0, "ExternFlag"=0, "DataLen"=0, "Data"=[], "Reserved"=[]} ("Send"), "ID"=w1130, "RemoteFlag"=w1136, "ExternFlag"=w1135, "DataLen"=w1140, "Data"=w1131) -> (w1137:T6)
            n469 = Build Array(w1137) -> (w1138:T6[])
            n470 = Unbundle By Name(w1133) -> ("DevType"=w1142:T5, "DevIndex"=w1141:u32, "CanIndex"=w1139:T4)
            n471 = call "VCI_Transmit.vi"("Buffer"=w1138, "CANIndex"=w1139, "DevIndex"=w1141, "DevType"=w1142) -> ()  [unwired: 1 in, 7 out]
          }
          event "T3_R": Value Change {
            w1157 = u8 0 items=["数据帧", "遥控帧"]
            w1156 = u8 0 items=["标准帧", "扩展帧"]
            # "地址"
            n472 = event-data() -> ()  [unwired: 2 out]
            n473 = property on="电机ID" class="CmbBox"() -> ("Value"=w1166:string)  [unwired: 2 in, 2 out]
            n474 = Scan From String(format string="%x" ("格式字符串"), input string=w1166, default 1=u8 0) -> (output 1=w1169:u8)  [unwired: 2 in, 3 out]
            n475 = call "Demo_MakeData.vi"("DataString"="66") -> ("Data"=w1152:u8[], "DataLen"=w1161:u8)  [unwired: 9 out]
            n476 = Add(x=u32 48, y=w1169) -> (x+y=w1151:u32)
            n477 = Bundle By Name(cluster=T6 {"ID"=0, "TimeStamp"=0, "TimeFlag"=0, "SendType"=0, "RemoteFlag"=0, "ExternFlag"=0, "DataLen"=0, "Data"=[], "Reserved"=[]} ("Send"), "ID"=w1151, "RemoteFlag"=w1157, "ExternFlag"=w1156, "DataLen"=w1161, "Data"=w1152) -> (w1158:T6)
            n478 = Build Array(w1158) -> (w1159:T6[])
            n479 = Unbundle By Name(w1154) -> ("DevType"=w1163:T5, "DevIndex"=w1162:u32, "CanIndex"=w1160:T4)
            n480 = call "VCI_Transmit.vi"("Buffer"=w1159, "CANIndex"=w1160, "DevIndex"=w1162, "DevType"=w1163) -> ()  [unwired: 1 in, 7 out]
          }
          event "T4_R": Value Change {
            w1188 = u8 0 items=["数据帧", "遥控帧"]
            w1189 = u8 0 items=["标准帧", "扩展帧"]
            # "地址"
            n481 = event-data() -> ()  [unwired: 2 out]
            n482 = property on="电机ID" class="CmbBox"() -> ("Value"=w1179:string)  [unwired: 2 in, 2 out]
            n483 = Scan From String(format string="%x" ("格式字符串"), input string=w1179, default 1=u8 0) -> (output 1=w1176:u8)  [unwired: 2 in, 3 out]
            n484 = call "Demo_MakeData.vi"("DataString"="67") -> ("Data"=w1173:u8[], "DataLen"=w1184:u8)  [unwired: 9 out]
            n485 = Add(x=u32 48, y=w1176) -> (x+y=w1174:u32)
            n486 = Bundle By Name(cluster=T6 {"ID"=0, "TimeStamp"=0, "TimeFlag"=0, "SendType"=0, "RemoteFlag"=0, "ExternFlag"=0, "DataLen"=0, "Data"=[], "Reserved"=[]} ("Send"), "ID"=w1174, "RemoteFlag"=w1188, "ExternFlag"=w1189, "DataLen"=w1184, "Data"=w1173) -> (w1187:T6)
            n487 = Build Array(w1187) -> (w1186:T6[])
            n488 = Unbundle By Name(w1175) -> ("DevType"=w1182:T5, "DevIndex"=w1183:u32, "CanIndex"=w1185:T4)
            n489 = call "VCI_Transmit.vi"("Buffer"=w1186, "CANIndex"=w1185, "DevIndex"=w1183, "DevType"=w1182) -> ()  [unwired: 1 in, 7 out]
          }
          event "保存": Value Change {
            w1216 = "-"
            n490 = event-data() -> ()  [unwired: 2 out]
            n491 = Get Date/Time String(want seconds? (F)=TRUE) -> (date string=w1196:string, time string=w1217:string)  [unwired: 2 in]
            n492 = Search and Replace String(input string=w1196, search string="/", replace string="-") -> (result string=w1202:string)  [unwired: 5 in, 3 out]
            n493 = Search and Replace String(input string=w1217, search string=":", replace string="-") -> (result string=w1214:string)  [unwired: 5 in, 3 out]
            n494 = property on="保存_S" class="Bool (严格)"() -> ("Value"=w1208:bool)  [unwired: 2 in, 2 out]
            n495 = Search and Replace String(input string=w1202, search string="/", replace string="-") -> (result string=w1197:string)  [unwired: 5 in, 3 out]
            n496 = Search and Replace String(input string=w1214, search string=":", replace string="-") -> (result string=w1215:string)  [unwired: 5 in, 3 out]
            n497 = Not(x=w1208) -> (.not. x?=w1204:bool)
            n498 = property on="保存_S" class="Bool (严格)"("Value"=w1204) -> ()  [unwired: 2 in, 2 out]
            n499 = Concatenate Strings("D:\\PMSM\\", w1197, w1216, w1215, w1216, "电机数据存储", ".txt") -> (w1194:string)
            n500 = Select(t=w1194, s=w1204, f="") -> (s? t:f=w1209:string)
            n501 = String To Path(string=w1209) -> (path=w1195:path)
            n502 = local write "存储路径"(w1195) -> ()
          }
          event "Close": Value Change {
            w1229 = T10 1 items=["OK"=1, "ERROR1"=0, "ERROR2"=-1] ("y")
            n503 = event-data() -> ()  [unwired: 2 out]
            n504 = Unbundle By Name(w1233) -> ("DevType"=w1232:T5, "DevIndex"=w1231:u32)
            n505 = call "VCI_CloseDevice.vi"("DevIndex"=w1231, "DevType"=w1232) -> ("Return Val"=w1230:T10)  [unwired: 1 in, 8 out]
            n506 = Equal?(x=w1230, y=w1229) -> (x = y?=w1227:bool)
            n507 = Not(x=w1227) -> (.not. x?=w1223:bool)
            n508 = Bundle By Name(cluster=cluster{"CANOpen":bool} {"CANOpen"=FALSE} ("事件数据"), "CANOpen"=w1223) -> (w1222:cluster{"CANOpen":bool})
            n509 = Bundle By Name(cluster=w1228, "Open"=w1223) -> (w1226:cluster{"Open":bool, "SendCnt":u32})
            n510 = local write "Open"(w1223) -> ()
            n511 = Generate User Event(user event=w1225, event data cluster=w1222) -> ()  [unwired: 1 in, 2 out]
          }
          event User Event {
            w1244 = u8 0
            w1243 = u8 2
            n512 = event-data() -> ("CANOpen"=w1237:bool)  [unwired: 1 out]
            "Open" <- w1237
            n513 = Not(x=w1237) -> (.not. x?=w1238:bool)
            n514 = Select(t=w1243, s=w1237, f=w1244) -> (s? t:f=w1236:u8)
            n515 = Select(t=w1244, s=w1237, f=w1243) -> (s? t:f=w1235:u8)
            n516 = property class="VI"("Front Panel.Closeable"=w1238) -> ()  [unwired: 2 in, 2 out]
            n517 = property on="Close" class="Bool"("DisabledEnum"=w1235) -> ()  [unwired: 2 in, 2 out]
            n518 = property on="ID" class="DigNum (严格)"("DisabledEnum"=w1235) -> ()  [unwired: 2 in, 2 out]
            n519 = property on="Data" class="Str"("DisabledEnum"=w1235) -> ()  [unwired: 2 in, 2 out]
            n520 = property on="Format" class="Ring (严格)"("DisabledEnum"=w1235) -> ()  [unwired: 2 in, 2 out]
            n521 = property on="Type" class="Ring (严格)"("DisabledEnum"=w1235) -> ()  [unwired: 2 in, 2 out]
            n522 = property on="Send" class="Bool"("DisabledEnum"=w1235) -> ()  [unwired: 2 in, 2 out]
            n523 = Select(t=enum16{"Init", "Wait", "Run", "Exit"}."Run", s=w1237, f=enum16{"Init", "Wait", "Run", "Exit"}."Wait") -> (s? t:f=w1240:enum16{"Init", "Wait", "Run", "Exit"})
            n524 = property on="Fliter" class="Ring (严格)"("DisabledEnum"=w1236) -> ()  [unwired: 2 in, 2 out]
            n525 = property on="DevType" class="Ring (严格)"("DisabledEnum"=w1236) -> ()  [unwired: 2 in, 2 out]
            n526 = property on="Channel" class="Ring (严格)"("DisabledEnum"=w1236) -> ()  [unwired: 2 in, 2 out]
            n527 = property on="AccCode" class="DigNum (严格)"("DisabledEnum"=w1236) -> ()  [unwired: 2 in, 2 out]
            n528 = property on="AccMask" class="DigNum (严格)"("DisabledEnum"=w1236) -> ()  [unwired: 2 in, 2 out]
            n529 = property on="InitFlag" class="Ring (严格)"("DisabledEnum"=w1236) -> ()  [unwired: 2 in, 2 out]
            n530 = property on="Mode" class="Ring (严格)"("DisabledEnum"=w1236) -> ()  [unwired: 2 in, 2 out]
            n531 = property on="kBaudRate" class="Ring (严格)"("DisabledEnum"=w1236) -> ()  [unwired: 2 in, 2 out]
            n532 = property on="电机ID_W" class="Bool"("DisabledEnum"=w1235) -> ()  [unwired: 2 in, 2 out]
            n533 = property on="监测_W" class="Bool"("DisabledEnum"=w1235) -> ()  [unwired: 2 in, 2 out]
            n534 = property on="模式_W" class="Bool"("DisabledEnum"=w1235) -> ()  [unwired: 2 in, 2 out]
            n535 = property on="模式_R" class="Bool"("DisabledEnum"=w1235) -> ()  [unwired: 2 in, 2 out]
            n536 = property on="设定位置_W" class="Bool"("DisabledEnum"=w1235) -> ()  [unwired: 2 in, 2 out]
            n537 = property on="设定位置_R" class="Bool"("DisabledEnum"=w1235) -> ()  [unwired: 2 in, 2 out]
            n538 = property on="设定速度_W" class="Bool"("DisabledEnum"=w1235) -> ()  [unwired: 2 in, 2 out]
            n539 = property on="设定速度_R" class="Bool"("DisabledEnum"=w1235) -> ()  [unwired: 2 in, 2 out]
            n540 = property on="设定电流_W" class="Bool"("DisabledEnum"=w1235) -> ()  [unwired: 2 in, 2 out]
            n541 = property on="设定电流_R" class="Bool"("DisabledEnum"=w1235) -> ()  [unwired: 2 in, 2 out]
            n542 = property on="保存" class="Bool"("DisabledEnum"=w1235) -> ()  [unwired: 2 in, 2 out]
            n543 = property on="Direction_W" class="Bool"("DisabledEnum"=w1235) -> ()  [unwired: 2 in, 2 out]
            n544 = property on="I_EN_W" class="Bool"("DisabledEnum"=w1235) -> ()  [unwired: 2 in, 2 out]
            n545 = property on="W_EN_W" class="Bool"("DisabledEnum"=w1235) -> ()  [unwired: 2 in, 2 out]
            n546 = property on="速度环KI_W" class="Bool"("DisabledEnum"=w1235) -> ()  [unwired: 2 in, 2 out]
            n547 = property on="加速度_W" class="Bool"("DisabledEnum"=w1235) -> ()  [unwired: 2 in, 2 out]
            n548 = property on="T1_W" class="Bool"("DisabledEnum"=w1235) -> ()  [unwired: 2 in, 2 out]
            n549 = property on="T2_W" class="Bool"("DisabledEnum"=w1235) -> ()  [unwired: 2 in, 2 out]
            n550 = property on="T3_W" class="Bool"("DisabledEnum"=w1235) -> ()  [unwired: 2 in, 2 out]
            n551 = property on="DATA_SAVE_W" class="Bool"("DisabledEnum"=w1235) -> ()  [unwired: 2 in, 2 out]
            n552 = property on="监测周期_W" class="Bool"("DisabledEnum"=w1235) -> ()  [unwired: 2 in, 2 out]
            n553 = property on="看门狗_W" class="Bool"("DisabledEnum"=w1235) -> ()  [unwired: 2 in, 2 out]
            n554 = property on="Direction_R" class="Bool"("DisabledEnum"=w1235) -> ()  [unwired: 2 in, 2 out]
            n555 = property on="I_EN_R" class="Bool"("DisabledEnum"=w1235) -> ()  [unwired: 2 in, 2 out]
            n556 = property on="W_EN_R" class="Bool"("DisabledEnum"=w1235) -> ()  [unwired: 2 in, 2 out]
            n557 = property on="速度环KI_R" class="Bool"("DisabledEnum"=w1235) -> ()  [unwired: 2 in, 2 out]
            n558 = property on="加速度_R" class="Bool"("DisabledEnum"=w1235) -> ()  [unwired: 2 in, 2 out]
            n559 = property on="T1_R" class="Bool"("DisabledEnum"=w1235) -> ()  [unwired: 2 in, 2 out]
            n560 = property on="T2_R" class="Bool"("DisabledEnum"=w1235) -> ()  [unwired: 2 in, 2 out]
            n561 = property on="T3_R" class="Bool"("DisabledEnum"=w1235) -> ()  [unwired: 2 in, 2 out]
            n562 = property on="监测周期_R" class="Bool"("DisabledEnum"=w1235) -> ()  [unwired: 2 in, 2 out]
            n563 = property on="看门狗周期_W" class="Bool"("DisabledEnum"=w1235) -> ()  [unwired: 2 in, 2 out]
            n564 = property on="看门狗周期_R" class="Bool"("DisabledEnum"=w1235) -> ()  [unwired: 2 in, 2 out]
            n565 = property on="减速度_R" class="Bool"("DisabledEnum"=w1235) -> ()  [unwired: 2 in, 2 out]
            n566 = property on="减速度_W" class="Bool"("DisabledEnum"=w1235) -> ()  [unwired: 2 in, 2 out]
            n567 = property on="T4_W" class="Bool"("DisabledEnum"=w1235) -> ()  [unwired: 2 in, 2 out]
            n568 = property on="T4_R" class="Bool"("DisabledEnum"=w1235) -> ()  [unwired: 2 in, 2 out]
            n569 = property on="电机校准_W" class="Bool"("DisabledEnum"=w1235) -> ()  [unwired: 2 in, 2 out]
            n570 = property on="W1_W" class="Bool"("DisabledEnum"=w1235) -> ()  [unwired: 2 in, 2 out]
            n571 = property on="W1_R" class="Bool"("DisabledEnum"=w1235) -> ()  [unwired: 2 in, 2 out]
            n572 = property on="W2_W" class="Bool"("DisabledEnum"=w1235) -> ()  [unwired: 2 in, 2 out]
            n573 = property on="W2_R" class="Bool"("DisabledEnum"=w1235) -> ()  [unwired: 2 in, 2 out]
            n574 = property on="W3_W" class="Bool"("DisabledEnum"=w1235) -> ()  [unwired: 2 in, 2 out]
            n575 = property on="W3_R" class="Bool"("DisabledEnum"=w1235) -> ()  [unwired: 2 in, 2 out]
            n576 = property on="W4_W" class="Bool"("DisabledEnum"=w1235) -> ()  [unwired: 2 in, 2 out]
            n577 = property on="W4_R" class="Bool"("DisabledEnum"=w1235) -> ()  [unwired: 2 in, 2 out]
          }
        }
        "数组" <- w150
        "CAN ID" <- w149
      }
      frame "Exit" {
        n578 = Release Queue(queue=w1255) -> ()  [unwired: 1 in, 4 out]
        n579 = Unregister For Events(event registration refnum=w1254) -> (error out=w1253:errorcluster)  [unwired: 1 in]
        n580 = Destroy User Event(user event=w1252, error in=w1253) -> ()  [unwired: 1 out]
        n581 = Unbundle By Name(w1251) -> ("Open"=w1250:bool)
        n582 = case shown="真" w1250 {
          tunnel: w1249 -> [_ w1259]
          frame False {
          }
          frame True {
            n583 = Unbundle By Name(w1259) -> ("DevType"=w1258:T5, "DevIndex"=w1257:u32)
            n584 = call "VCI_CloseDevice.vi"("DevIndex"=w1257, "DevType"=w1258) -> ()  [unwired: 1 in, 9 out]
          }
        }
        n585 = local write "RcvEnable"(FALSE ("RcvEnable")) -> ()
      }
    }
  }
  n586 = while "数据更新线程" {
    tunnel: w9 -> [w1265]
    shift-right: [w1260] -> _
    shift-left: u32 0 ("RecvCnt") -> [w1261]
    stop <- w1264 stop-if-true
    n587 = Dequeue Element(queue=w1265) -> (element=w1263:T7, timed out?=w1262:bool, error out=w1264:errorcluster)  [unwired: 2 in, 1 out]
    n588 = case shown="假" w1262 {
      tunnel: w1263 -> [w1275 _]
      tunnel: w1261 -> [w1269 w1668]
      tunnel: [w1268 w1668] -> w1260
      frame False {
        n589 = Array To Cluster(array=w1275) -> (cluster=w1277:T12)
        n590 = Unbundle By Name(w1277) -> ("[0]"=w1276:T13)
        n591 = Increment(x=w1269) -> (x+1=w1268:u32)
        "sCnt" <- w1268
        n592 = Unbundle By Name(w1276) -> ("VCI_CAN_OBJ"=w1274:T6)  [unwired: 3 out]
        n593 = Unbundle By Name(w1274) -> ("ID"=w1272:u32, "Data"=w1273:u8[])  [unwired: 7 out]
        "CAN STD_ID" <- w1272
        n594 = And(x=w1272, y=u32 15) -> (x .and. y?=→"电机ID_R":u32)
        n595 = And(x=w1272, y=u32 240) -> (x .and. y?=w1267:u32)
        n596 = case shown="40" w1267 {
          tunnel: w1273 -> [_ w1283]
          frame 0, Default {
          }
          frame 64 {
            n597 = local read "存储路径"() -> (w1279:path)
            n598 = local read "保存_S"() -> (w1280:bool)
            n599 = Index Array(array=w1283, index=0) -> (element=w1282:u8)
            n600 = case shown="6A" w1282 {
              tunnel: w1283 -> [_ w1308 w1317 w1330 w1341 w1348 w1366 w1386 w1410 w1427 w1447 w1460 w1485 w1504 w1521 w1525 w1532 _ w1540 w1550 w1556 w1569 w1572 w1582 w1592 w1602 _ w1612 w1618 w1627 w1630 w1636 w1642 w1648 w1651 w1654 w1657 w1663]
              tunnel: [_ _ _ _ _ _ w1354 w1376 w1399 w1425 w1442 w1459 w1474 w1498 _ _ _ _ _ _ _ _ _ _ _ _ _ _ _ _ _ _ _ _ _ _ _ _] -> w1278
              frame 0, Default {
              }
              frame 1 {
                n601 = Array To Cluster(array=w1308) -> (cluster=w1309:T14)
                n602 = Unbundle By Name(w1309) -> ("Data[1]"=w1311:u8, "Data[2]"=w1312:u8)  [unwired: 1 out]
                n603 = Join Numbers(hi=w1311, lo=w1312) -> ((hi.lo)=w1310:u16)
                n604 = To Unsigned Word Integer(number=w1310) -> (unsigned 16bit integer=→"看门狗周期_回":u16)
              }
              frame 32 {
                n605 = Array To Cluster(array=w1317) -> (cluster=w1318:T14)
                n606 = Unbundle By Name(w1318) -> ("Data[1]"=w1316:u8)  [unwired: 1 out]
                n607 = To Unsigned Byte Integer(number=w1316) -> (unsigned 8bit integer=w1313:u8)
                n608 = Number To Hexadecimal String(1:2, 2:w1313) -> (0:w1314:string)
                n609 = property on="模式_回" class="CmbBox"("Value"=w1314) -> ()  [unwired: 2 in, 2 out]
              }
              frame 33 {
                n610 = Array To Cluster(array=w1330) -> (cluster=w1332:T14)
                n611 = Unbundle By Name(w1332) -> ("Data[1]"=w1331:u8)  [unwired: 1 out]
                n612 = To Unsigned Byte Integer(number=w1331) -> (unsigned 8bit integer=w1329:u8)
                n613 = Number To Boolean Array(number=w1329) -> (Boolean array=w1328:bool[])
                n614 = Array To Cluster(array=w1328) -> (cluster=w1327:T15)
                n615 = Unbundle(w1327) -> ("Boolean array[0]"=→"warn0":bool, "Boolean array[1]"=→"warn1":bool, "Boolean array[2]"=→"高温":bool, "Boolean array[3]"=→"warn3":bool, "Boolean array[4]"=→"warn4":bool, "Boolean array[5]"=→"warn5":bool, "Boolean array[6]"=→"warn6":bool, "Boolean array[7]"=→"warn7":bool)
              }
              frame 34 {
                n616 = Array To Cluster(array=w1341) -> (cluster=w1346:T14)
                n617 = Unbundle By Name(w1346) -> ("Data[1]"=w1345:u8)  [unwired: 1 out]
                n618 = To Unsigned Byte Integer(number=w1345) -> (unsigned 8bit integer=w1344:u8)
                n619 = Number To Boolean Array(number=w1344) -> (Boolean array=w1343:bool[])
                n620 = Array To Cluster(array=w1343) -> (cluster=w1342:T15)
                n621 = Unbundle(w1342) -> ("Boolean array[0]"=→"低压":bool, "Boolean array[1]"=→"高压":bool, "Boolean array[2]"=→"高温":bool, "Boolean array[3]"=→"ERRO3":bool, "Boolean array[4]"=→"ERRO4":bool, "Boolean array[5]"=→"ERRO5":bool, "Boolean array[6]"=→"ERRO6":bool, "Boolean array[7]"=→"ERRO7":bool)
              }
              frame 35 {
                n622 = Array To Cluster(array=w1348) -> (cluster=w1349:T14)
                n623 = Unbundle By Name(w1349) -> ("Data[1]"=w1351:u8, "Data[2]"=w1352:u8)  [unwired: 1 out]
                n624 = Join Numbers(hi=w1351, lo=w1352) -> ((hi.lo)=w1350:u16)
                n625 = To Unsigned Word Integer(number=w1350) -> (unsigned 16bit integer=→"监测周期_回":u16)
              }
              frame 49 {
                w1355 = 0.0054931640625
                w1368 = 8
                n626 = Array To Cluster(array=w1366) -> (cluster=w1372:T14)
                n627 = Unbundle By Name(w1372) -> ("Data[1]"=w1360:u8, "Data[2]"=w1361:u8, "Data[3]"=w1362:u8, "Data[4]"=w1363:u8, "Data[5]"=w1359:u8, "Data[6]"=w1358:u8)  [unwired: 1 out]
                n628 = Join Numbers(hi=w1359, lo=w1358) -> ((hi.lo)=w1357:u16)
                n629 = To Unsigned Word Integer(number=w1360) -> (unsigned 16bit integer=w1375:u16)
                n630 = To Unsigned Word Integer(number=w1362) -> (unsigned 16bit integer=w1371:u16)
                n631 = To Word Integer(number=w1357) -> (16bit integer=w1356:i16)
                n632 = Rotate(1:w1375, 2:w1368) -> (0:w1374:u16)
                n633 = Rotate(1:w1371, 2:w1368) -> (0:w1370:u16)
                n634 = Add(x=w1374, y=w1361) -> (x+y=w1373:u16)
                n635 = Add(x=w1370, y=w1363) -> (x+y=w1369:u16)
                n636 = Multiply(x=w1373, y=w1355) -> (x*y=w1365:dbl)
                "机械角度" <- w1365
                n637 = Multiply(x=w1369, y=w1355) -> (x*y=w1364:dbl)
                "电气角度" <- w1364
                n638 = Divide(x=w1356, y=1.0) -> (x/y=w1353:dbl)
                "转速" <- w1353
                "转速" <- w1353
                n639 = Build Array(w1365, w1364, w1353) -> (w1354:dbl[])
              }
              frame 50 {
                w1387 = i16 1024
                w1388 = 8
                n640 = Array To Cluster(array=w1386) -> (cluster=w1395:T14)
                n641 = Unbundle By Name(w1395) -> ("Data[1]"=w1385:u8, "Data[2]"=w1384:u8, "Data[3]"=w1383:u8, "Data[4]"=w1382:u8, "Data[5]"=w1381:u8, "Data[6]"=w1380:u8)  [unwired: 1 out]
                n642 = To Word Integer(number=w1385) -> (16bit integer=w1398:i16)
                n643 = To Word Integer(number=w1381) -> (16bit integer=w1391:i16)
                n644 = To Word Integer(number=w1383) -> (16bit integer=w1394:i16)
                n645 = Rotate(1:w1398, 2:w1388) -> (0:w1397:i16)
                n646 = Rotate(1:w1391, 2:w1388) -> (0:w1390:i16)
                n647 = Rotate(1:w1394, 2:w1388) -> (0:w1393:i16)
                n648 = Add(x=w1397, y=w1384) -> (x+y=w1396:i16)
                n649 = Add(x=w1390, y=w1380) -> (x+y=w1389:i16)
                n650 = Add(x=w1393, y=w1382) -> (x+y=w1392:i16)
                n651 = Divide(x=w1396, y=w1387) -> (x/y=w1379:dbl)
                "A电流" <- w1379
                "波形图表1" <- w1379
                n652 = Divide(x=w1389, y=w1387) -> (x/y=w1377:dbl)
                "C电流" <- w1377
                "波形图表3" <- w1377
                n653 = Divide(x=w1392, y=w1387) -> (x/y=w1378:dbl)
                "B电流" <- w1378
                "波形图表2" <- w1378
                n654 = Build Array(w1379, w1378, w1377) -> (w1376:dbl[])
              }
              frame 51 {
                w1412 = i16 256
                w1411 = 8
                n655 = Array To Cluster(array=w1410) -> (cluster=w1419:T14)
                n656 = Unbundle By Name(w1419) -> ("Data[1]"=w1409:u8, "Data[2]"=w1408:u8, "Data[3]"=w1407:u8, "Data[4]"=w1406:u8, "Data[5]"=w1405:u8, "Data[6]"=w1404:u8)  [unwired: 1 out]
                n657 = To Unsigned Word Integer(number=w1409) -> (unsigned 16bit integer=w1422:u16)
                n658 = To Word Integer(number=w1407) -> (16bit integer=w1418:i16)
                n659 = To Word Integer(number=w1405) -> (16bit integer=w1415:i16)
                n660 = Rotate(1:w1422, 2:w1411) -> (0:w1421:u16)
                n661 = Rotate(1:w1418, 2:w1411) -> (0:w1417:i16)
                n662 = Rotate(1:w1415, 2:w1411) -> (0:w1414:i16)
                n663 = Add(x=w1421, y=w1408) -> (x+y=w1420:u16)
                n664 = Add(x=w1417, y=w1406) -> (x+y=w1416:i16)
                n665 = Add(x=w1414, y=w1404) -> (x+y=w1413:i16)
                n666 = Divide(x=w1420, y=i16 1024) -> (x/y=w1402:dbl)
                "供电电压" <- w1402
                n667 = Divide(x=w1416, y=w1412) -> (x/y=w1401:dbl)
                "Ialfa" <- w1401
                n668 = Divide(x=w1413, y=w1412) -> (x/y=w1400:dbl)
                "Ibeta" <- w1400
                n669 = Build Array(w1402, w1401, w1400) -> (w1399:dbl[])
              }
              frame 52 {
                w1426 = i16 256
                w1432 = 8
                n670 = Array To Cluster(array=w1427) -> (cluster=w1436:T14)
                n671 = Unbundle By Name(w1436) -> ("Data[1]"=w1431:u8, "Data[2]"=w1430:u8, "Data[3]"=w1429:u8, "Data[4]"=w1428:u8)  [unwired: 1 out]
                n672 = To Word Integer(number=w1431) -> (16bit integer=w1439:i16)
                n673 = To Word Integer(number=w1429) -> (16bit integer=w1435:i16)
                n674 = Rotate(1:w1439, 2:w1432) -> (0:w1438:i16)
                n675 = Rotate(1:w1435, 2:w1432) -> (0:w1434:i16)
                n676 = Add(x=w1438, y=w1430) -> (x+y=w1437:i16)
                n677 = Add(x=w1434, y=w1428) -> (x+y=w1433:i16)
                n678 = Divide(x=w1437, y=w1426) -> (x/y=w1424:dbl)
                "Iqnow" <- w1424
                n679 = Divide(x=w1433, y=w1426) -> (x/y=w1423:dbl)
                "Idnow" <- w1423
                n680 = Build Array(w1424, w1423) -> (w1425:dbl[])
              }
              frame 53 {
                w1449 = i16 1024
                w1448 = 8
                n681 = Array To Cluster(array=w1447) -> (cluster=w1453:T14)
                n682 = Unbundle By Name(w1453) -> ("Data[1]"=w1446:u8, "Data[2]"=w1445:u8, "Data[3]"=w1444:u8, "Data[4]"=w1443:u8)  [unwired: 1 out]
                n683 = To Word Integer(number=w1446) -> (16bit integer=w1456:i16)
                n684 = To Word Integer(number=w1444) -> (16bit integer=w1452:i16)
                n685 = Rotate(1:w1456, 2:w1448) -> (0:w1455:i16)
                n686 = Rotate(1:w1452, 2:w1448) -> (0:w1451:i16)
                n687 = Add(x=w1455, y=w1445) -> (x+y=w1454:i16)
                n688 = Add(x=w1451, y=w1443) -> (x+y=w1450:i16)
                n689 = Divide(x=w1454, y=w1449) -> (x/y=w1441:dbl)
                "Uq" <- w1441
                n690 = Divide(x=w1450, y=w1449) -> (x/y=w1440:dbl)
                "Ud" <- w1440
                n691 = Build Array(w1441, w1440) -> (w1442:dbl[])
              }
              frame 54 {
                w1466 = i16 1024
                w1465 = 8
                n692 = Array To Cluster(array=w1460) -> (cluster=w1470:T14)
                n693 = Unbundle By Name(w1470) -> ("Data[1]"=w1464:u8, "Data[2]"=w1463:u8, "Data[3]"=w1462:u8, "Data[4]"=w1461:u8)  [unwired: 1 out]
                n694 = To Word Integer(number=w1464) -> (16bit integer=w1473:i16)
                n695 = To Word Integer(number=w1462) -> (16bit integer=w1469:i16)
                n696 = Rotate(1:w1473, 2:w1465) -> (0:w1472:i16)
                n697 = Rotate(1:w1469, 2:w1465) -> (0:w1468:i16)
                n698 = Add(x=w1472, y=w1463) -> (x+y=w1471:i16)
                n699 = Add(x=w1468, y=w1461) -> (x+y=w1467:i16)
                n700 = Divide(x=w1471, y=w1466) -> (x/y=w1458:dbl)
                "Ualfa" <- w1458
                n701 = Divide(x=w1467, y=w1466) -> (x/y=w1457:dbl)
                "Ubate" <- w1457
                n702 = Build Array(w1458, w1457) -> (w1459:dbl[])
              }
              frame 55 {
                w1487 = u16 0
                w1486 = 8
                n703 = Array To Cluster(array=w1485) -> (cluster=w1494:T14)
                n704 = Unbundle By Name(w1494) -> ("Data[1]"=w1479:u8, "Data[2]"=w1480:u8, "Data[3]"=w1481:u8, "Data[4]"=w1482:u8, "Data[5]"=w1483:u8, "Data[6]"=w1484:u8, "Data[7]"=w1475:u8)  [unwired: 1 out]
                "sector" <- w1475
                n705 = To Word Integer(number=w1479) -> (16bit integer=w1497:i16)
                n706 = To Word Integer(number=w1481) -> (16bit integer=w1493:i16)
                n707 = To Word Integer(number=w1483) -> (16bit integer=w1490:i16)
                n708 = Rotate(1:w1497, 2:w1486) -> (0:w1496:i16)
                n709 = Rotate(1:w1493, 2:w1486) -> (0:w1492:i16)
                n710 = Rotate(1:w1490, 2:w1486) -> (0:w1489:i16)
                n711 = Add(x=w1496, y=w1480) -> (x+y=w1495:i16)
                n712 = Add(x=w1492, y=w1482) -> (x+y=w1491:i16)
                n713 = Add(x=w1489, y=w1484) -> (x+y=w1488:i16)
                n714 = Subtract ("减")(x=w1495, y=w1487) -> (x-y=w1478:u16)
                "PWM1" <- w1478
                n715 = Subtract ("减")(x=w1491, y=w1487) -> (x-y=w1477:u16)
                "PWM2" <- w1477
                n716 = Subtract ("减")(x=w1488, y=w1487) -> (x-y=w1476:u16)
                "PWM3" <- w1476
                n717 = Build Array(w1478, w1477, w1476, w1475) -> (w1474:u16[])
              }
              frame 56 {
                n718 = Array Subset(array=w1504, index=1, length=4) -> (w1501:u8[])
                n719 = Type Cast(type=2097152, x=w1501) -> (*(type *) &x=w1499:i32)
                "Sin" <- w1499
                "Cosin" <- w1499
                n720 = Build Array(w1499, w1499) -> (w1498:i32[])
              }
              frame 57 {
                n721 = Array To Cluster(array=w1521) -> (cluster=w1522:cluster{"Data[0]":u8, "Data[1]":u8})
                n722 = Unbundle By Name(w1522) -> ("Data[1]"=w1513:u8)  [unwired: 1 out]
                n723 = And(x=w1513, y=u8 56) -> (x .and. y?=w1516:u8)
                n724 = And(x=w1513, y=u8 192) -> (x .and. y?=w1519:u8)
                n725 = And(x=w1513, y=u8 7) -> (x .and. y?=w1510:u8)
                n726 = Logical Shift(y=i16 -3, x=w1516) -> (x << y=w1512:u8)
                n727 = Logical Shift(y=i16 -6, x=w1519) -> (x << y=w1508:u8)
                n728 = Divide(x=w1512, y=u8 10) -> (x/y=w1507:dbl)
                n729 = Divide(x=w1510, y=u8 100) -> (x/y=w1506:dbl)
                n730 = Compound Arithmetic op=ADD(w1508, w1507, w1506) -> (→"版本号":dbl)
              }
              frame 58 {
                n731 = Array To Cluster(array=w1525) -> (cluster=w1530:T14)
                n732 = Unbundle By Name(w1530) -> ("Data[1]"=w1528:u8, "Data[2]"=w1527:u8)  [unwired: 1 out]
                n733 = Join Numbers(hi=w1528, lo=w1527) -> ((hi.lo)=w1529:u16)
                n734 = To Unsigned Word Integer(number=w1529) -> (unsigned 16bit integer=w1526:u16)
                n735 = Multiply(x=w1526, y=0.0054931640625) -> (x*y=w1524:dbl)
                n736 = property on="机械角度" class="DigNum (严格)"("Value"=w1524) -> ()  [unwired: 2 in, 2 out]
              }
              frame 59 {
                n737 = Array To Cluster(array=w1532) -> (cluster=w1538:T14)
                n738 = Unbundle By Name(w1538) -> ("Data[1]"=w1536:u8, "Data[2]"=w1535:u8)  [unwired: 1 out]
                n739 = Join Numbers(hi=w1536, lo=w1535) -> ((hi.lo)=w1537:u16)
                n740 = To Word Integer(number=w1537) -> (16bit integer=w1534:i16)
                n741 = Divide(x=w1534, y=i16 1) -> (x/y=w1531:dbl)
                n742 = property on="转速" class="DigNum (严格)"("Value"=w1531) -> ()  [unwired: 2 in, 2 out]
              }
              frame 62 {
              }
              frame 60 {
                n743 = Array To Cluster(array=w1540) -> (cluster=w1546:T14)
                n744 = Unbundle By Name(w1546) -> ("Data[1]"=w1544:u8, "Data[2]"=w1543:u8)  [unwired: 1 out]
                n745 = Join Numbers(hi=w1544, lo=w1543) -> ((hi.lo)=w1545:u16)
                n746 = To Word Integer(number=w1545) -> (16bit integer=w1542:i16)
                n747 = Divide(x=w1542, y=i16 256) -> (x/y=w1539:dbl)
                n748 = property on="Iqnow" class="DigNum (严格)"("Value"=w1539) -> ()  [unwired: 2 in, 2 out]
              }
              frame 61 {
                n749 = Array To Cluster(array=w1550) -> (cluster=w1554:T14)
                n750 = Unbundle By Name(w1554) -> ("Data[1]"=w1552:u8, "Data[2]"=w1551:u8)  [unwired: 1 out]
                n751 = Join Numbers(hi=w1552, lo=w1551) -> ((hi.lo)=w1553:u16)
                n752 = To Word Integer(number=w1553) -> (16bit integer=w1549:i16)
                n753 = Divide(x=w1549, y=i16 4) -> (x/y=→"温度":dbl)
              }
              frame 64 {
                n754 = Array To Cluster(array=w1556) -> (cluster=w1561:T14)
                n755 = Unbundle By Name(w1561) -> ("Data[1]"=w1557:u8, "Data[2]"=w1558:u8)  [unwired: 1 out]
                n756 = To Unsigned Word Integer(number=w1557) -> (unsigned 16bit integer=w1564:u16)
                n757 = Rotate(1:w1564, 2:8) -> (0:w1563:u16)
                n758 = Add ("加")(x=w1563, y=w1558) -> (x+y=w1562:u16)
                n759 = Divide(x=w1562, y=u16 256) -> (x/y=→"设定位置_回":dbl)
              }
              frame 65 {
                n760 = Array To Cluster(array=w1569) -> (cluster=w1570:T14)
                n761 = Unbundle By Name(w1570) -> ("Data[1]"=w1567:u8, "Data[2]"=w1566:u8)  [unwired: 1 out]
                n762 = Join Numbers(hi=w1567, lo=w1566) -> ((hi.lo)=w1568:u16)
                n763 = To Word Integer(number=w1568) -> (16bit integer=→"设定速度_回":i16)
              }
              frame 66 {
                n764 = Array To Cluster(array=w1572) -> (cluster=w1577:T14)
                n765 = Unbundle By Name(w1577) -> ("Data[1]"=w1573:u8, "Data[2]"=w1574:u8)  [unwired: 1 out]
                n766 = To Word Integer(number=w1573) -> (16bit integer=w1580:i16)
                n767 = Rotate(1:w1580, 2:8) -> (0:w1579:i16)
                n768 = Add ("加")(x=w1579, y=w1574) -> (x+y=w1578:i16)
                n769 = Divide(x=w1578, y=u16 256) -> (x/y=→"设定电流_回":dbl)
              }
              frame 81 {
                n770 = Array To Cluster(array=w1582) -> (cluster=w1587:T14)
                n771 = Unbundle By Name(w1587) -> ("Data[1]"=w1583:u8, "Data[2]"=w1584:u8)  [unwired: 1 out]
                n772 = To Unsigned Word Integer(number=w1583) -> (unsigned 16bit integer=w1590:u16)
                n773 = Rotate(1:w1590, 2:8) -> (0:w1589:u16)
                n774 = Add ("加")(x=w1589, y=w1584) -> (x+y=w1588:u16)
                n775 = Divide(x=w1588, y=u16 256) -> (x/y=→"速度环KI_回":dbl)
              }
              frame 82 {
                n776 = Array To Cluster(array=w1592) -> (cluster=w1597:T14)
                n777 = Unbundle By Name(w1597) -> ("Data[1]"=w1593:u8, "Data[2]"=w1594:u8)  [unwired: 1 out]
                n778 = To Unsigned Word Integer(number=w1593) -> (unsigned 16bit integer=w1600:u16)
                n779 = Rotate(1:w1600, 2:8) -> (0:w1599:u16)
                n780 = Add ("加")(x=w1599, y=w1594) -> (x+y=w1598:u16)
                n781 = Divide(x=w1598, y=u16 8) -> (x/y=→"加速度_回":dbl)
              }
              frame 83 {
                n782 = Array To Cluster(array=w1602) -> (cluster=w1607:T14)
                n783 = Unbundle By Name(w1607) -> ("Data[1]"=w1603:u8, "Data[2]"=w1604:u8)  [unwired: 1 out]
                n784 = To Unsigned Word Integer(number=w1603) -> (unsigned 16bit integer=w1610:u16)
                n785 = Rotate(1:w1610, 2:8) -> (0:w1609:u16)
                n786 = Add ("加")(x=w1609, y=w1604) -> (x+y=w1608:u16)
                n787 = Divide(x=w1608, y=u16 8) -> (x/y=→"减速度_回":dbl)
              }
              frame 86 {
              }
              frame 99 {
                n788 = Array To Cluster(array=w1612) -> (cluster=w1616:T14)
                n789 = Unbundle By Name(w1616) -> ("Data[1]"=w1614:u8, "Data[2]"=w1613:u8)  [unwired: 1 out]
                n790 = Join Numbers(hi=w1614, lo=w1613) -> ((hi.lo)=w1615:u16)
                n791 = To Unsigned Word Integer(number=w1615) -> (unsigned 16bit integer=→"W4":u16)
              }
              frame 98 {
                n792 = Array To Cluster(array=w1618) -> (cluster=w1622:T14)
                n793 = Unbundle By Name(w1622) -> ("Data[1]"=w1620:u8, "Data[2]"=w1619:u8)  [unwired: 1 out]
                n794 = Join Numbers(hi=w1620, lo=w1619) -> ((hi.lo)=w1621:u16)
                n795 = To Unsigned Word Integer(number=w1621) -> (unsigned 16bit integer=→"W3":u16)
              }
              frame 100 {
                n796 = Array To Cluster(array=w1627) -> (cluster=w1628:T14)
                n797 = Unbundle By Name(w1628) -> ("Data[1]"=w1625:u8, "Data[2]"=w1624:u8)  [unwired: 1 out]
                n798 = Join Numbers(hi=w1625, lo=w1624) -> ((hi.lo)=w1626:u16)
                n799 = To Unsigned Word Integer(number=w1626) -> (unsigned 16bit integer=→"T1":u16)
              }
              frame 101 {
                n800 = Array To Cluster(array=w1630) -> (cluster=w1634:T14)
                n801 = Unbundle By Name(w1634) -> ("Data[1]"=w1632:u8, "Data[2]"=w1631:u8)  [unwired: 1 out]
                n802 = Join Numbers(hi=w1632, lo=w1631) -> ((hi.lo)=w1633:u16)
                n803 = To Unsigned Word Integer(number=w1633) -> (unsigned 16bit integer=→"T2":u16)
              }
              frame 102 {
                n804 = Array To Cluster(array=w1636) -> (cluster=w1640:T14)
                n805 = Unbundle By Name(w1640) -> ("Data[1]"=w1638:u8, "Data[2]"=w1637:u8)  [unwired: 1 out]
                n806 = Join Numbers(hi=w1638, lo=w1637) -> ((hi.lo)=w1639:u16)
                n807 = To Unsigned Word Integer(number=w1639) -> (unsigned 16bit integer=→"T3":u16)
              }
              frame 103 {
                n808 = Array To Cluster(array=w1642) -> (cluster=w1646:T14)
                n809 = Unbundle By Name(w1646) -> ("Data[1]"=w1644:u8, "Data[2]"=w1643:u8)  [unwired: 1 out]
                n810 = Join Numbers(hi=w1644, lo=w1643) -> ((hi.lo)=w1645:u16)
                n811 = To Unsigned Word Integer(number=w1645) -> (unsigned 16bit integer=→"T4":u16)
              }
              frame 104 {
                n812 = Array To Cluster(array=w1648) -> (cluster=w1649:T14)
                n813 = Unbundle By Name(w1649) -> ("Data[1]"=→"电流使能":u8)  [unwired: 1 out]
              }
              frame 105 {
                n814 = Array To Cluster(array=w1651) -> (cluster=w1652:T14)
                n815 = Unbundle By Name(w1652) -> ("Data[1]"=→"功率使能":u8)  [unwired: 1 out]
              }
              frame 106 {
                n816 = Array To Cluster(array=w1654) -> (cluster=w1655:T14)
                n817 = Unbundle By Name(w1655) -> ("Data[1]"=→"方向":u8)  [unwired: 1 out]
              }
              frame 96 {
                n818 = Array To Cluster(array=w1657) -> (cluster=w1656:T14)
                n819 = Unbundle By Name(w1656) -> ("Data[1]"=w1658:u8, "Data[2]"=w1659:u8)  [unwired: 1 out]
                n820 = Join Numbers(hi=w1658, lo=w1659) -> ((hi.lo)=w1661:u16)
                n821 = To Unsigned Word Integer(number=w1661) -> (unsigned 16bit integer=→"W1":u16)
              }
              frame 97 {
                n822 = Array To Cluster(array=w1663) -> (cluster=w1667:T14)
                n823 = Unbundle By Name(w1667) -> ("Data[1]"=w1665:u8, "Data[2]"=w1664:u8)  [unwired: 1 out]
                n824 = Join Numbers(hi=w1665, lo=w1664) -> ((hi.lo)=w1666:u16)
                n825 = To Unsigned Word Integer(number=w1666) -> (unsigned 16bit integer=→"W2":u16)
              }
            }
            n826 = case shown="真" w1280 {
              tunnel: w1279 -> [_ w1290]
              tunnel: w1278 -> [_ w1288]
              frame False {
              }
              frame True {
                n827 = Array Size(array=w1288) -> (size(s)=w1289:i32)
                n828 = Open/Create/Replace File(file path (use dialog)=w1290, operation (0:open)=T11."open or create") -> (refnum out=w1298:refnum<file>, error out=w1287:errorcluster)  [unwired: 4 in, 1 out]
                n829 = for {
                  N: w1289 -> [_]
                  shift-right: [w1306] -> w1295
                  shift-left: "" -> [w1303]
                  tunnel: w1288 -> [w1301]
                  i -> [w1302]
                  # "浮点文本存储"
                  # "2-14"
                  n830 = Index Array(array=w1301, index=w1302) -> (element=w1300:dbl)
                  n831 = Number To Fractional String(number=w1300) -> (F-format string=w1305:string)  [unwired: 3 in]
                  n832 = Concatenate Strings(w1303, w1305, "\t") -> (w1306:string)
                }
                n833 = Set File Position(refnum=w1298, from (0:start)=u16 1, error in=w1287) -> (refnum out=w1297:refnum<file>, error out=w1286:errorcluster)  [unwired: 1 in]
                n834 = Concatenate Strings(w1295, "\r") -> (w1293:string)
                n835 = Write to Text File(file (use dialog)=w1297, text=w1293, error in=w1286) -> (refnum out=w1296:refnum<file>, error out=w1285:errorcluster)  [unwired: 1 in, 1 out]
                n836 = Close File(refnum=w1296, error in=w1285) -> (error out=w1284:errorcluster)  [unwired: 1 out]
                n837 = call <vilib>:"Clear Errors.vi"("error in (no error)"=w1284) -> ()  [unwired: 6 in, 1 out]
              }
            }
          }
        }
      }
      frame True {
      }
    }
  }
  n838 = while "接收线程" {
    tunnel: w9 -> [w1671]
    shift-right: [w1669] -> _
    shift-left: u32 0 ("RecvCnt") -> [w1670]
    stop <- "RcvEnable" continue-if-true
    n839 = local read "Open"() -> (w1672:bool)
    n840 = case shown="真" w1672 {
      tunnel: w1671 -> [_ w1679]
      tunnel: w1670 -> [w1674 w1678]
      tunnel: [w1674 w1677] -> w1669
      frame False {
        # "CAN未打开，延时50ms"
        n841 = Wait (ms)(milliseconds to wait=u32 50 ("等待时间（毫秒）")) -> ()  [unwired: 1 out]
      }
      frame True {
        n842 = local read "DevType"() -> (w1683:T5)
        n843 = local read "Channel"() -> (w1676:T4)
        n844 = call "VCI_Receive.vi"("CANIndex"=w1676, "DevIndex"=u32 0, "DevType"=w1683) -> ("Recieve"=w1680:T6[])  [unwired: 3 in, 5 out]
        n845 = Empty Array?(array=w1680) -> (empty?=w1681:bool)
        n846 = case shown="假" w1681 {
          tunnel: w1679 -> [w1690 _]
          tunnel: w1680 -> [w1685 _]
          tunnel: [w1689 _] -> _
          tunnel: w1678 -> [w1687 w1702]
          tunnel: [w1686 w1702] -> w1677
          tunnel: w1676 -> [w1688 _]
          frame False {
            n847 = Array Size(array=w1685) -> (size(s)=w1684:i32)
            n848 = for {
              N: w1684 -> [_]
              tunnel: w1690 -> [w1701]
              tunnel: [w1699] -> w1689 mode=indexing
              tunnel: w1685 -> [w1694]
              tunnel: w1688 -> [w1698]
              shift-right: [w1695] -> w1686
              shift-left: w1687 -> [w1696]
              i -> [w1692]
              n849 = Array Subset(array=w1694, index=w1692, length=1) -> (w1693:T6[])
              n850 = Increment(x=w1696) -> (x+1=w1695:u32)
              n851 = call "Demo_MakeDispBuff.vi"("Channel"=w1698, "Type"=enum16{"接收", "发送"}."接收", "OBJs"=w1693) -> ("Buffer"=w1700:T7)
              n852 = Enqueue Element(queue=w1701, element=w1700) -> (error out=w1699:errorcluster)  [unwired: 1 in, 3 out]
            }
            "RecvCnt" <- w1686
          }
          frame True {
          }
        }
      }
    }
  }
  n853 = control-ref of="本应用程序"() -> (w6:refnum<vi>)
  n854 = invoke class="VI" method="FP.Close"(error in=w4) -> (error out=w3:errorcluster)  [unwired: 2 in, 2 out]
  n855 = property class="App"(reference=w6) -> ("App.Kind"=w5:T16)  [unwired: 1 in, 2 out]
  n856 = case shown="\"Development System\"" w5 {
    tunnel: w3 -> [_ _]
    frame "invalid app kind", Default {
      n857 = Quit LabVIEW() -> ()  [unwired: 1 out]
    }
    frame "Development System" {
    }
  }
